vi "Main.vi"() -> ()   [LabVIEW 2019]
uses:
  Controls/Main-state.ctl
  Controls/eFGV States.ctl
  Controls/FGV States.ctl
  Controls/Global - IP Address.vi
  Controls/Global - Handle.vi
  Controls/Global - Device.vi
  Controls/Global - Comport.vi
  Controls/Global - Channel.vi
  Controls/Global - Unit.vi
  Controls/Global - Done.vi
  Controls/Global - ADC.vi
  Controls/Global - Data UDP.vi
  Controls/Global - PID.vi
  Controls/Global - System.vi
  Controls/Global - Test.vi
  Controls/UDP - Command.ctl
  <vilib>/Utility/miscctls.llb/LVRectTypeDef.ctl
  Controls/UDP - Status.ctl
  Controls/UDP - Event.ctl
  Controls/Tab Button.ctl
  <vilib>/httpClient/LabVIEWHTTPClient.lvlib
  <vilib>/httpClient/POSTBuffer.vi
panel:
  out "Close Panel":T1
  in  "Path":path
  in  "Next":bool
  in  "Previous":bool
  in  "Tab Array":T2
  out "Event":string
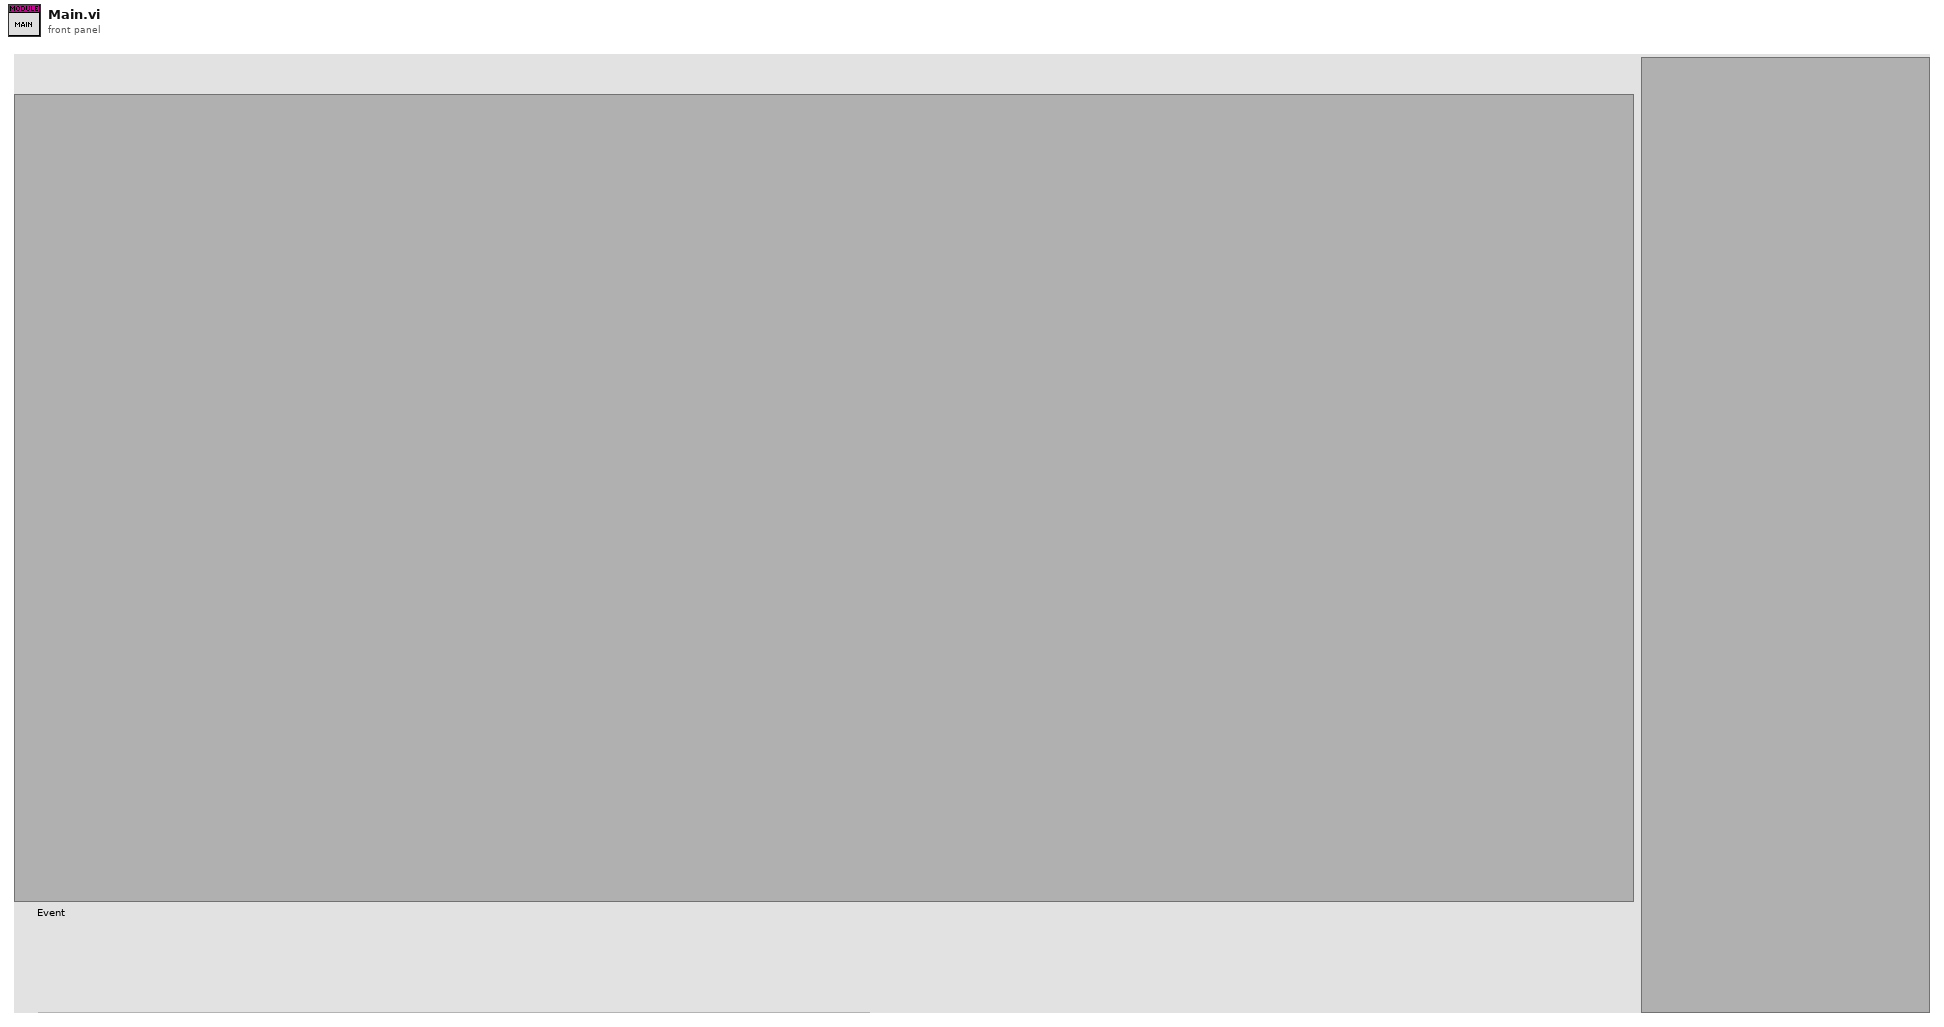
[diagram p1: front panel]
types:
  T1 = cluster{"String":string, "Cancel Button":bool, "OK Button":bool, "Bg":bool, "RunTest":refnum<vi>, "fileid":string}
  T2 = typedef "Tab Button.ctl" = cluster{"String":string, "Cancel Button":bool, "OK Button":bool, "Bg":bool, "RunTest":refnum<vi>, "fileid":string, "Stop":bool, "Run":bool, "Status":string}[]
  T3 = typedef "Main-state.ctl" = enum16{"Init", "Run modules", "Idle", "Change page", "Manual Control", "NewTest", "sidepanel", "Event", "Emergency", "Exit"}
  T4 = enum32{"Invalid", "Standard", "Closed", "Hidden", "Minimized", "Maximized"}
  T5 = enum32{"invalid app kind", "Development System", "Run Time System", "Student Edition", "Embedded LabVIEW", "Evaluation", "Custom"}
  T6 = cluster{"Module Ref":refnum<vi>[], "Side Name":string, "pin":bool, "FileId":string}
  T7 = typedef "FGV States.ctl" = enum16{"Read", "Write"}
  T8 = typedef "eFGV States.ctl" = enum16{"Init", "Read", "Write", "Exit"}
  T9 = enum16{"New Test", "Test Plan", "Job Record", "Instrument", "Machine", "Station", "Machine Control"}
  T10 = typedef "LVRectTypeDef.ctl" = cluster{"Left":i16, "Top":i16, "Right":i16, "Bottom":i16}
  T11 = typedef "UDP - Command.ctl" = enum16{"Stop", "Jog Up", "Jog Down", "Ramp Up", "Ramp Down", "PID Target", "PID Ramp", "Disp Run", "Read Ch Data", "Zero Channel", "Zero Disp", "Read Sensor", "Write Sensor", "Read ADC", "Write ADC", "Read PID", "Write PID", "Read Test", "Write Test", "Read System", "Write System", "Read Datalog", "Read Datalog Sensor"}
  T12 = cluster{"String":string, "Cancel Button":bool, "OK Button":bool, "Bg":bool, "RunTest":refnum<vi>, "fileid":string, "Stop":bool, "Run":bool, "Status":string}
  T13 = cluster{"String":string, "Cancel Button":bool, "OK Button":bool, "Bg":bool, "RunTest":refnum<vi>, "fileid":string, "Stop":bool, "Run":bool, "Status":string}[]
  T14 = typedef "LabVIEWHTTPClient.lvlib/ClientHandle.ctl" = refnum<k1>
  T15 = cluster{"IP Address":string, "port":string, "UDP ref":refnum<k16>}[]
  T16 = typedef "UDP - Event.ctl" = u16
  T17 = typedef "UDP - Status.ctl" = u16
  T18 = cluster{"Channels":cluster{"Ch1":sgl, "Ch2":sgl, "Ch3":sgl, "Ch4":sgl, "Ch5":sgl, "Ch6":sgl, "Ch7":sgl, "Ch8":sgl, "Ch9":sgl, "Ch10":sgl, "Ch11":sgl, "Ch12":sgl, "Ch13":sgl, "Ch14":sgl, "Ch15":sgl, "Ch16":sgl}, "Event":T16, "Status":T17}[]
  T19 = cluster{"Ch1":sgl, "Ch2":sgl, "Ch3":sgl, "Ch4":sgl, "Ch5":sgl, "Ch6":sgl, "Ch7":sgl, "Ch8":sgl, "Ch9":sgl, "Ch10":sgl, "Ch11":sgl, "Ch12":sgl, "Ch13":sgl, "Ch14":sgl, "Ch15":sgl, "Ch16":sgl}
  T20 = cluster{"Target Load":sgl, "Target Disp":sgl, "Rate":sgl, "Speed":sgl}[]
  T21 = cluster{"Out Type":u8, "Inverse":u8, "Monitor":u8, "Reserve":u8, "ACC Time":u32, "Pulse Rev":u32, "Stroke":u32, "Auto Off":u32, "Gear Ratio":sgl, "Pitch":sgl, "Max Speed":u32, "Jog Speed":u32, "Disp Coff":sgl, "Max Load":u32}[]
  T22 = cluster{"SP":sgl, "PV":sgl, "kP":sgl, "kI":sgl, "kD":sgl, "FF":sgl, "Err Band":sgl, "Max":i32, "Min":i32, "Ts":u32, "Out":i32, "Mode":u8}[]
  T23 = cluster{"Active Ch":u8[], "Filter Type":u8, "Post Filter":u8[], "Gain":u8[], "FS":u16, "IntOC":u8, "IntFC":u8, "SysOC":u8, "Cofficient":dbl[], "K":dbl[], "Max":i32}[]
  T24 = cluster{"Name":string[], "Unit":string[], "Decimal Point":u8[], "Ch Log":u8[], "H Alarm":u8[], "L Alarm":u8[], "H Limit":sgl[], "L Limit":sgl[], "Filter":u8[], "Gain":u8[], "Calib Type":u32[]}[]
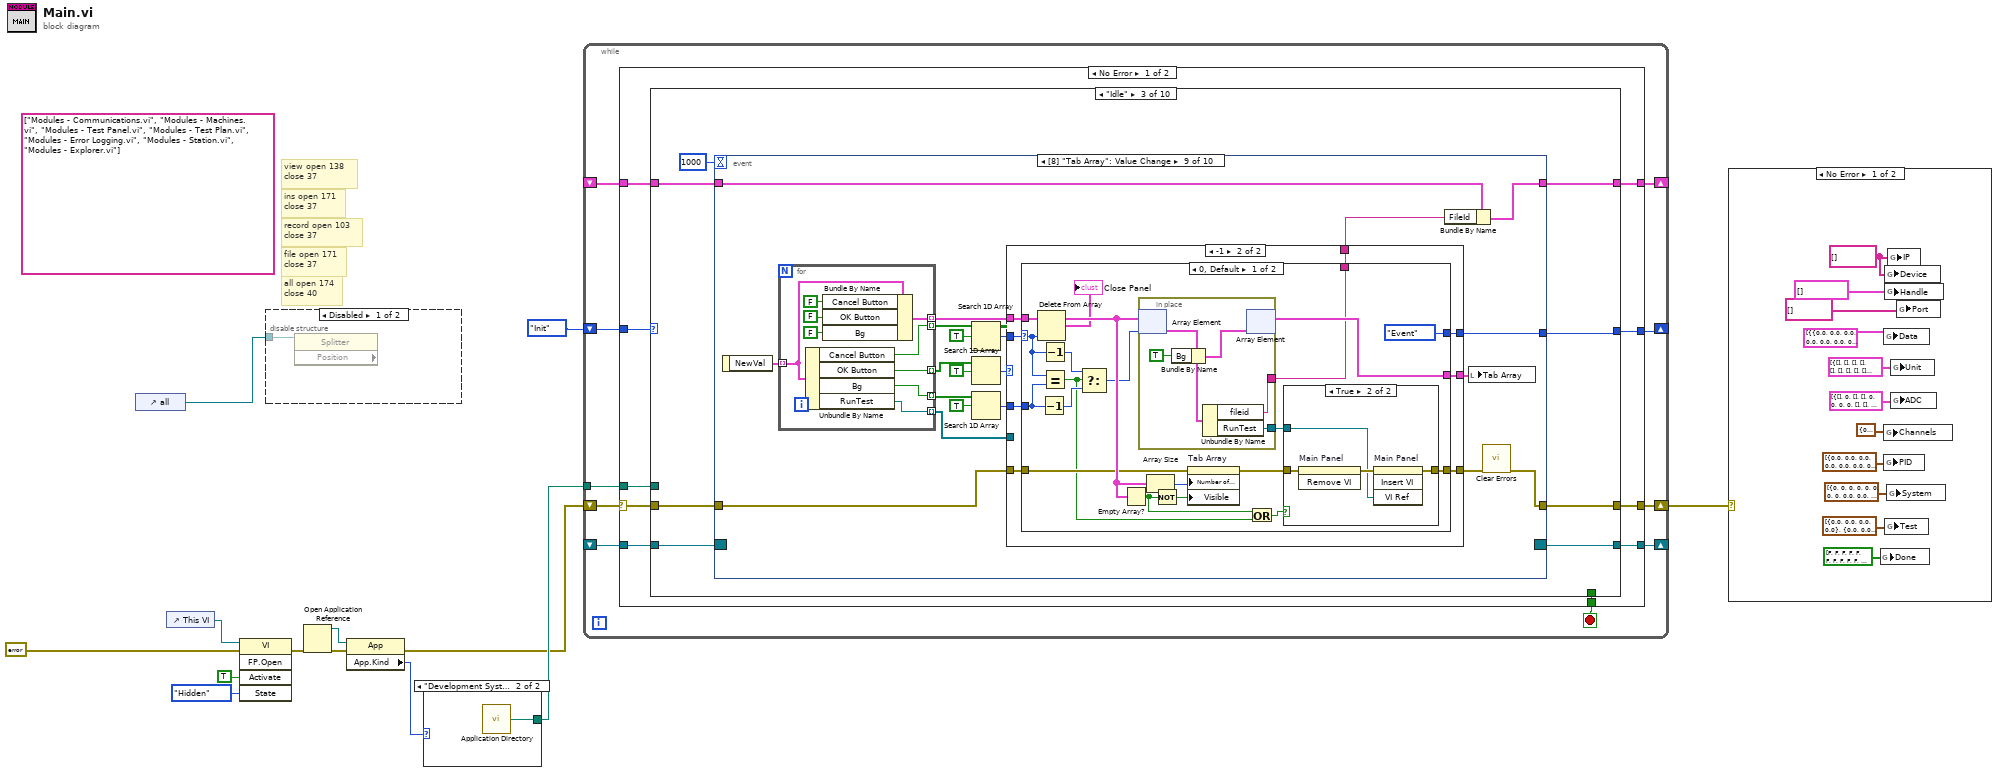
[diagram p0: block diagram]
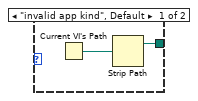
[diagram p2: hidden frame]
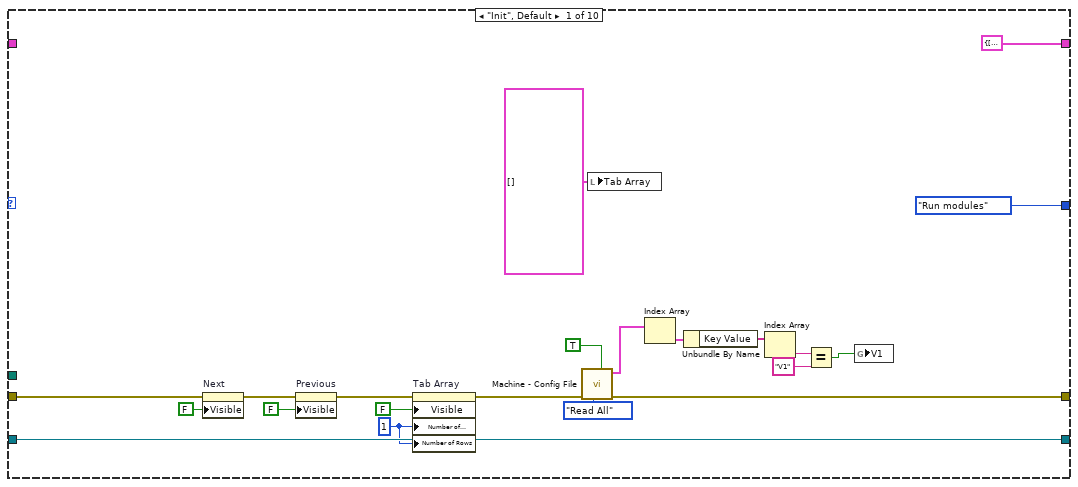
[diagram p4: hidden frame]
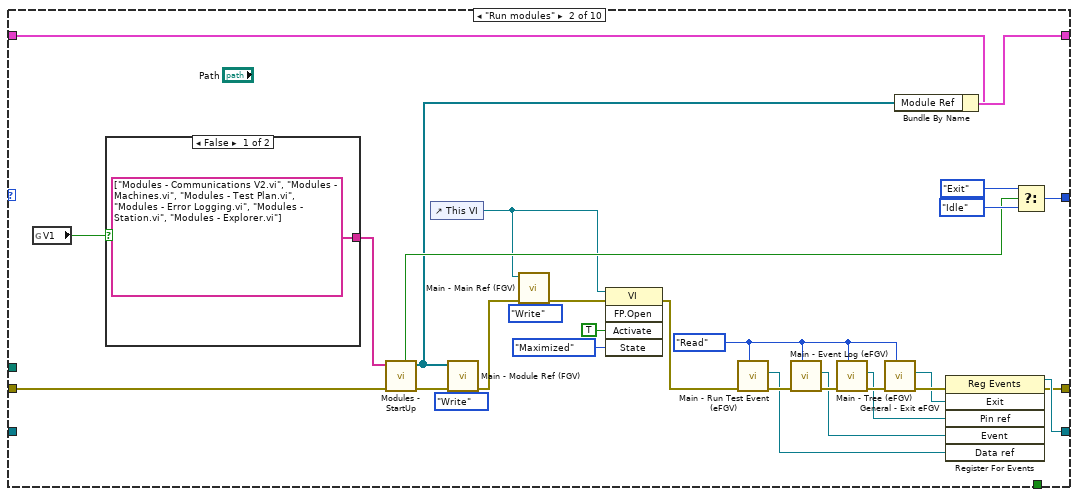
[diagram p5: hidden frame]
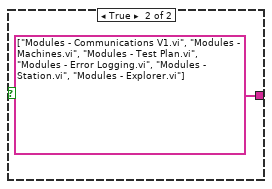
[diagram p6: hidden frame]
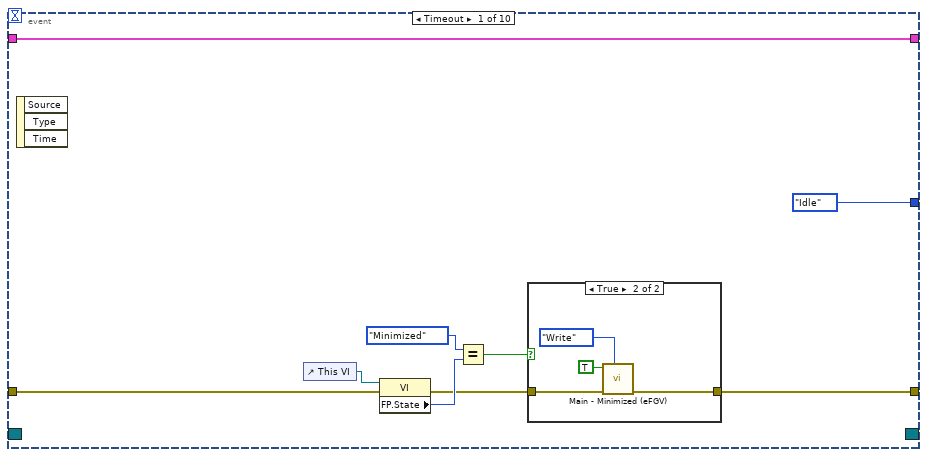
[diagram p7: hidden frame]
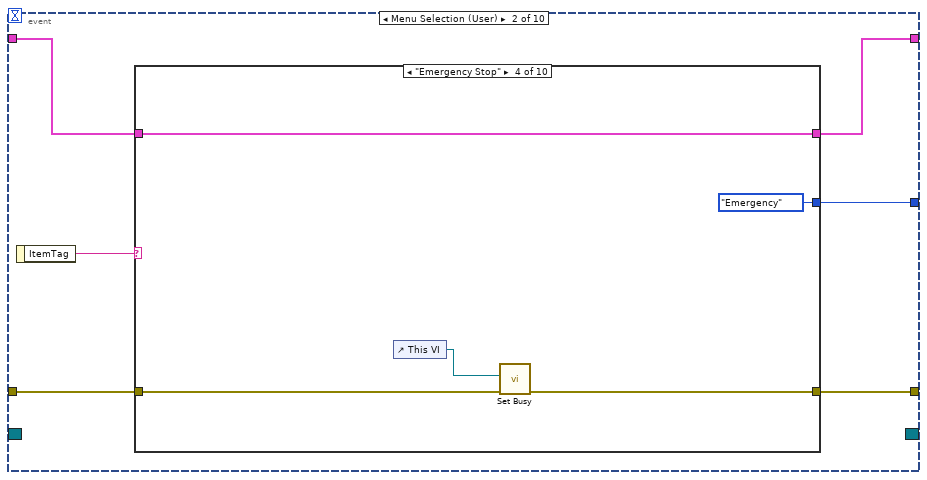
[diagram p9: hidden frame]
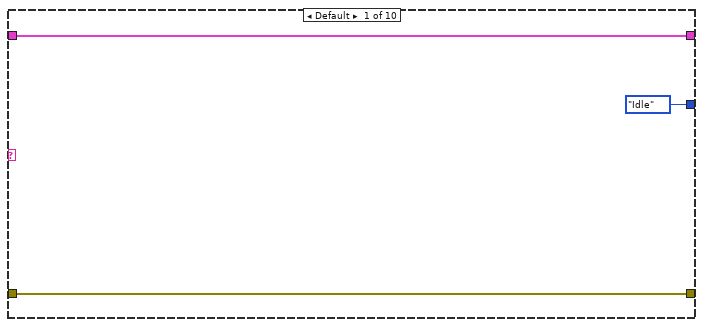
[diagram p10: hidden frame]
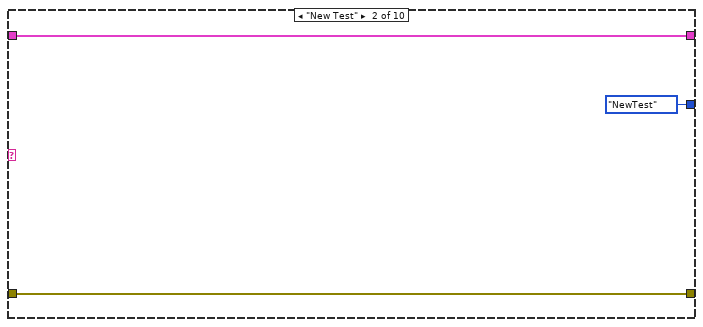
[diagram p11: hidden frame]
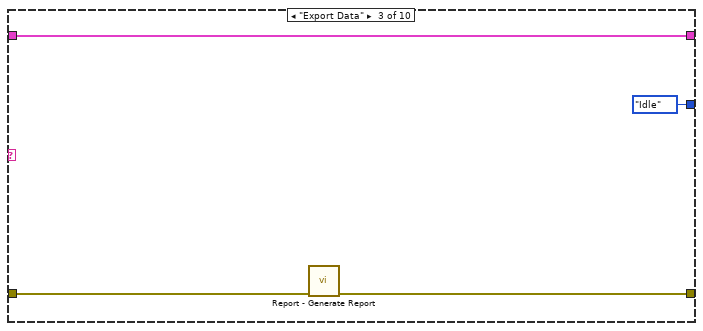
[diagram p12: hidden frame]
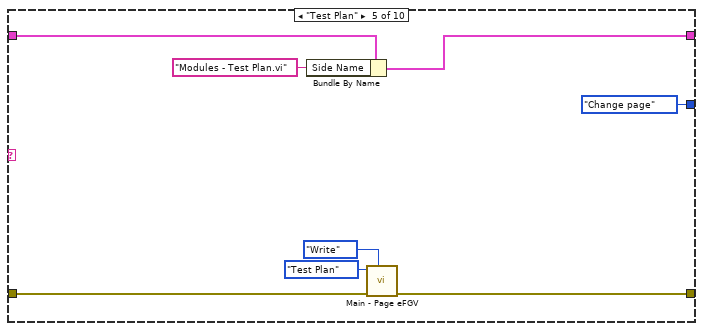
[diagram p13: hidden frame]
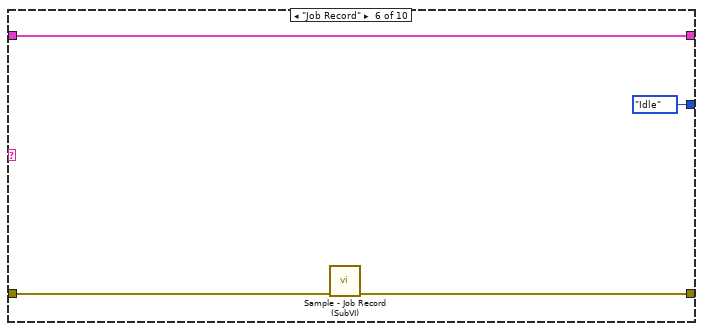
[diagram p14: hidden frame]
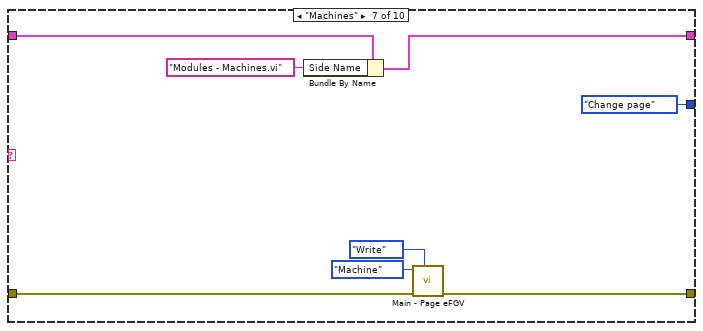
[diagram p15: hidden frame]
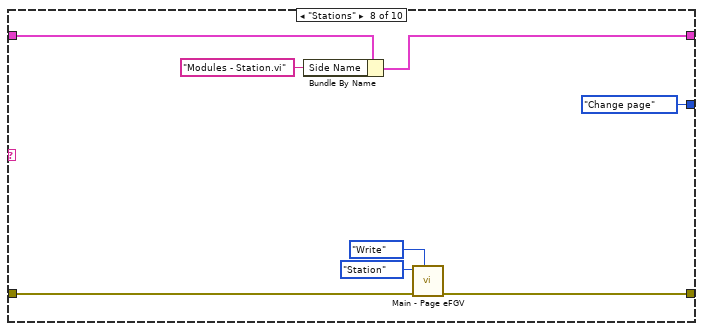
[diagram p16: hidden frame]
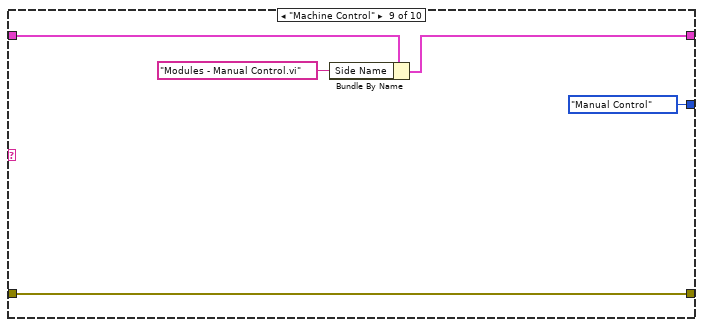
[diagram p17: hidden frame]
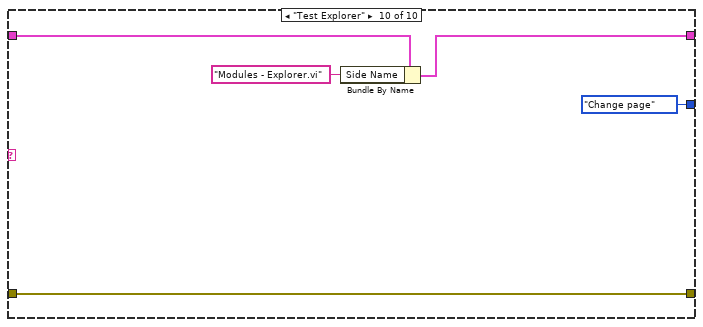
[diagram p18: hidden frame]
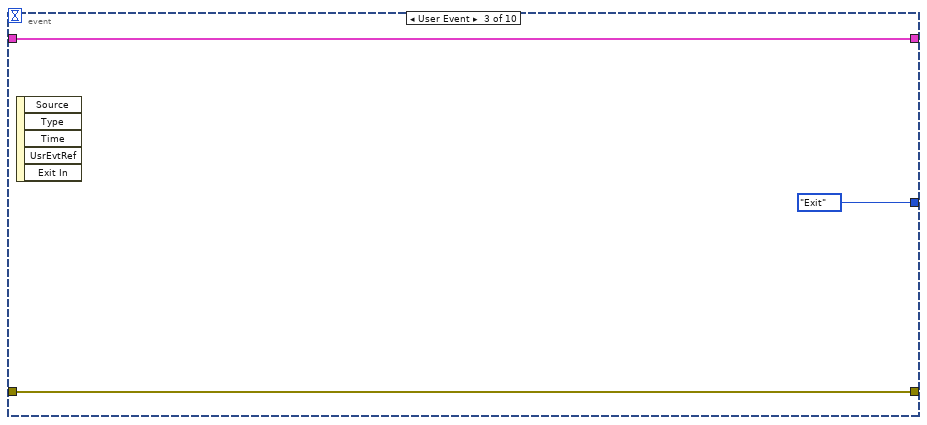
[diagram p19: hidden frame]
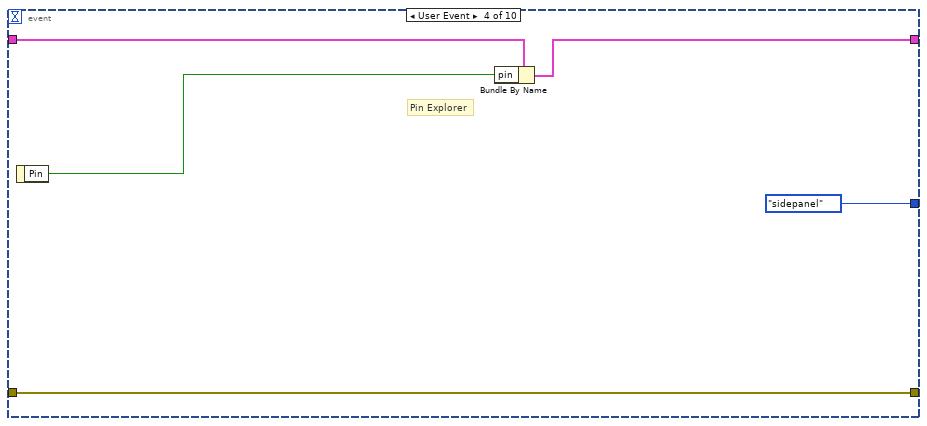
[diagram p20: hidden frame]
diagram:
  (unwired) string[] ["Modules - Communications.vi", "Modules - Machines.vi", "Modules - Test Panel.vi", "Modules - Test Plan.vi", "Modules - Error Logging.vi", "Modules - Station.vi", "Modules - Explorer.vi"]
  # "view open 138\nclose 37"
  # "record open 103\nclose 37"
  # "ins open 171\nclose 37"
  # "all open 174\nclose 40"
  # "file open 171\nclose 37"
  n1 = control-ref of="all"() -> (w1:refnum<vi>)
  n2 = control-ref of="This VI"() -> (w10:refnum<vi>)
  n3 = invoke class="VI" method="FP.Open"(reference=w10, error in=errorcluster {"status"=FALSE, "code"=0, "source"=""} ("error constant"), "Activate"=TRUE ("Activate?"), "State"=T4."Hidden") -> (error out=w5:errorcluster)  [unwired: 1 in, 4 out]
  n4 = disable-structure shown="Disabled" {
    disable-tunnel: w1 -> [w14 _]
    frame Disabled {
      n5 = property class="Splitter" props=["Position"](reference=w14) -> ()  [unwired: 1 in, 3 out]
    }
    frame Enabled {
    }
  }
  n6 = Open Application Reference(8:w5) -> (0:w7:errorcluster, 3:w6:refnum<vi>)  [unwired: 3 in]
  n7 = property class="App"(reference=w6, error in=w7) -> (error out=w2:errorcluster, "App.Kind"=w4:T5)  [unwired: 1 out]
  n8 = case shown="\"Development System\"" w4 {
    tunnel: [w15 w17] -> w3
    frame "invalid app kind", Default {
      n9 = Current VI's Path() -> (path=w16:path)
      n10 = Strip Path(path=w16) -> (stripped path=w15:path)  [unwired: 1 out]
    }
    frame "Development System" {
      n11 = call <vilib>:"Application Directory.vi"() -> ("Application Directory"=w17:path)
    }
  }
  n12 = while {
    shift-right: [w24] -> _
    shift-left: Main-state."Init" -> [w26]
    shift-right: [w25] -> w8
    shift-left: w2 -> [w27]
    shift-right: [w22] -> _
    shift-left: _ -> [w21]
    shift-right: [w20] -> _
    shift-left: _ -> [w19]
    tunnel: w3 -> [w18]
    stop <- w23 stop-if-true
    n13 = case shown="No Error" w27 {
      selector: w27 -> [w36 w640]
      tunnel: w26 -> [w37 _]
      tunnel: [w35 w637] -> w25
      tunnel: [w34 Main-state."Idle"] -> w24
      tunnel: [w33 _] -> w23
      tunnel: [w32 w639] -> w22
      tunnel: w21 -> [w31 w639]
      tunnel: [w30 w635] -> w20
      tunnel: w19 -> [w29 w635]
      tunnel: w18 -> [w28 _]
      frame No Error {
        n14 = case shown="\"Idle\"" w37 {
          tunnel: w36 -> [w53 w86 w97 w381 w415 w458 w478 w514 w575 w604]
          tunnel: [w46 w61 w98 w384 w420 w457 w481 w509 w572 w608] -> w35
          tunnel: [Main-state."Run modules" w81 w94 Main-state."Idle" Main-state."Idle" Main-state."Idle" Main-state."Idle" Main-state."Idle" Main-state."Idle" Main-state."Exit"] -> w34
          tunnel: [_ _ _ _ _ _ _ _ _ TRUE] -> w33
          tunnel: [T6 {"Module Ref"=[], "Side Name"="", "pin"=FALSE, "FileId"=""} w88 w95 w383 w424 w471 w480 w513 w577 T6 {"Module Ref"=[], "Side Name"="", "pin"=FALSE, "FileId"=""}] -> w32
          tunnel: w31 -> [_ w60 w96 w383 w424 w471 w480 w513 w577 w616]
          tunnel: [w57 w74 w91 w377 w425 w472 w483 w518 w578 w606] -> w30
          tunnel: w29 -> [w57 _ w92 w377 w425 w472 w483 w518 w578 w606]
          tunnel: w28 -> [_ _ _ _ w411 w465 _ _ _ _]
          frame "Init", Default {
            w50 = u32 1 ("Number of Columns")
            n15 = property on="Next" class="Bool"(error in=w53, "Visible"=FALSE) -> (error out=w54:errorcluster)  [unwired: 1 in, 1 out]
            n16 = property on="Previous" class="Bool"(error in=w54, "Visible"=FALSE) -> (error out=w52:errorcluster)  [unwired: 1 in, 1 out]
            n17 = property on="Tab Array" class="Arr"(error in=w52, "Visible"=FALSE, "Number of Columns"=w50, "Number of Rows"=w50) -> (error out=w47:errorcluster)  [unwired: 1 in, 1 out]
            n18 = call "Machine - Config File.vi"("Setting"=TRUE, "Action"=enum16{"Write", "Read", "Read All", "Remove"}."Read All", "error in (no error)"=w47) -> ("error out"=w46:errorcluster, "Value Out"=w42:cluster{"IP/SN":string, "Key Value":string[]}[])  [unwired: 7 in]
            n19 = local write "Tab Array"(T2 [] ("Array")) -> ()
            n20 = Index Array(array=w42) -> (element=w44:cluster{"IP/SN":string, "Key Value":string[]})  [unwired: 1 in]
            n21 = Unbundle By Name(w44) -> ("Key Value"=w43:string[])
            n22 = Index Array(array=w43) -> (element=w40:string)  [unwired: 1 in]
            n23 = Equal?(x=w40, y="V1") -> (x = y?=w38:bool)
            n24 = global write "Global - Data UDP.vi" "V1"(w38) -> ()
          }
          frame "Run modules" {
            w63 = eFGV_States."Read" ("Action")
            n25 = global read "Global - Data UDP.vi" "V1"() -> (w59:bool)
            n26 = case shown="False" w59 {
              tunnel: [string[] ["Modules - Communications V2.vi", "Modules - Machines.vi", "Modules - Test Plan.vi", "Modules - Error Logging.vi", "Modules - Station.vi", "Modules - Explorer.vi"] string[] ["Modules - Communications V1.vi", "Modules - Machines.vi", "Modules - Test Plan.vi", "Modules - Error Logging.vi", "Modules - Station.vi", "Modules - Explorer.vi"]] -> w87
              frame False {
              }
              frame True {
              }
            }
            n27 = call "Modules - StartUp.vi"("Error In"=w86, "List of Modules"=w87) -> ("Error Out"=w78:errorcluster, "Module Ref"=w77:refnum<vi>[], "Force Exit"=w80:bool)  [unwired: 7 in]
            n28 = control-ref of="This VI"() -> (w69:refnum<vi>)
            n29 = call "Main - Module Ref (FGV).vi"("Action"=FGV_States."Write", "error in"=w78, "Ref in"=w77) -> ("error out"=w71:errorcluster)  [unwired: 7 in, 1 out]
            n30 = call "Main - Main Ref (FGV).vi"("Action"=FGV_States."Write", "error in"=w71, "This VI"=w69) -> ("error out"=w70:errorcluster)  [unwired: 7 in, 1 out]
            n31 = invoke class="VI" method="FP.Open"(reference=w69, error in=w70, "Activate"=TRUE ("Activate?"), "State"=T4."Maximized") -> (error out=w65:errorcluster)  [unwired: 1 in, 4 out]
            n32 = call "Main - Run Test Event (eFGV).vi"("Action"=w63, "error in"=w65) -> ("error out"=w64:errorcluster, "Data ref"=w62:refnum<user-event>)  [unwired: 7 in, 1 out]
            n33 = call "Main - Event Log (eFGV).vi"("Action"=w63, "error in"=w64) -> ("error out"=w67:errorcluster, "Event"=w66:refnum<user-event>)  [unwired: 6 in, 2 out]
            n34 = call "Main - Tree (eFGV).vi"("Action"=w63, "error in"=w67) -> ("error out"=w73:errorcluster, "Pin ref"=w72:refnum<user-event>)  [unwired: 7 in, 1 out]
            n35 = call "General - Exit eFGV.vi"("eFGV States"=w63, "error in (no error)"=w73) -> ("error out"=w76:errorcluster, "Exit"=w75:refnum<user-event>)  [unwired: 7 in, 1 out]
            n36 = Bundle By Name(cluster=w60, "Module Ref"=w77) -> (w88:T6)
            n37 = register-events(error in=w76, w75, w72, w66, w62) -> (reference out=w74:refnum<event-registration>, error out=w61:errorcluster)  [unwired: 1 in]
            n38 = Select(t=Main-state."Exit", s=w80, f=Main-state."Idle") -> (s? t:f=w81:T3)
          }
          frame "Idle" {
            n39 = event shown="[8] \"Tab Array\": Value Change" {
              selector: w92 -> [_ _ _ _ _ _ _ _ _ _]
              dyn-events: [_ _ _ _ _ _ _ _ _ _] -> w91
              timeout: 1000 -> [_ _ _ _ _ _ _ _ _ _]
              tunnel: [w100 w118 w174 w179 w183 w186 w192 w213 w237 w324] -> w98
              tunnel: w97 -> [w104 w117 w174 w179 w183 w187 w191 w212 w240 w323]
              tunnel: w96 -> [w107 w114 w173 w176 w181 w189 w203 w224 w235 w331]
              tunnel: [w107 w113 w173 w177 w182 w189 w203 w224 w236 w331] -> w95
              tunnel: [Main-state."Idle" w115 Main-state."Exit" Main-state."sidepanel" Main-state."Event" Main-state."Exit" Main-state."Idle" Main-state."Idle" w233 Main-state."Idle"] -> w94
              event Timeout {
                n40 = event-data() -> ()  [unwired: 1 in, 3 out]
                n41 = control-ref of="This VI"() -> (w105:refnum<vi>)
                n42 = property class="VI"(reference=w105, error in=w104) -> (error out=w99:errorcluster, "FP.State"=w102:T4)  [unwired: 1 out]
                n43 = Equal?(x=T4."Minimized" ("Front Panel Window:State"), y=w102) -> (x = y?=w101:bool)
                n44 = case shown="True" w101 {
                  tunnel: [w108 w111] -> w100
                  tunnel: w99 -> [w108 w112]
                  frame False {
                  }
                  frame True {
                    n45 = call "Main - Minimized (eFGV).vi"("Action"=eFGV_States."Write", "error in"=w112, "Minimized In"=TRUE) -> ("error out"=w111:errorcluster)  [unwired: 6 in, 2 out]
                  }
                }
              }
              event Menu Selection (User) {
                n46 = event-data() -> ("ItemTag"=w116:string)  [unwired: 1 in]
                n47 = case shown="\"Emergency Stop\"" w116 {
                  tunnel: [w121 w124 w127 w131 w137 w143 w149 w157 w166 w171] -> w118
                  tunnel: w117 -> [w121 w124 w126 w130 w136 w142 w148 w156 w166 w171]
                  tunnel: [Main-state."Idle" Main-state."NewTest" Main-state."Idle" Main-state."Emergency" Main-state."Change page" Main-state."Idle" Main-state."Change page" Main-state."Change page" Main-state."Manual Control" Main-state."Change page"] -> w115
                  tunnel: [w119 w122 w125 w129 w135 w144 w147 w155 w164 w168] -> w113
                  tunnel: w114 -> [w119 w122 w125 w129 w134 w144 w146 w154 w163 w167]
                  frame Default {
                  }
                  frame "New Test" {
                  }
                  frame "Export Data" {
                    n48 = call "Report - Generate Report.vi"("error in"=w126) -> ("error out"=w127:errorcluster)  [unwired: 10 in]
                  }
                  frame "Emergency Stop" {
                    n49 = control-ref of="This VI"() -> (w132:refnum<vi>)
                    n50 = call <vilib>:"Set Busy.vi"("error in (no error)"=w130, "VI reference (current VI)"=w132) -> ("error out"=w131:errorcluster)  [unwired: 8 in, 1 out]
                  }
                  frame "Test Plan" {
                    n51 = Bundle By Name(cluster=w134, "Side Name"="Modules - Test Plan.vi") -> (w135:T6)
                    n52 = call "Main - Page eFGV.vi"("eFGV States"=eFGV_States."Write", "error in (no error)"=w136, "Page In"=T9."Test Plan") -> ("error out"=w137:errorcluster)  [unwired: 6 in, 2 out]
                  }
                  frame "Job Record" {
                    n53 = call "Sample - Job Record (SubVI).vi"("error in"=w142) -> ("error out"=w143:errorcluster)  [unwired: 10 in]
                  }
                  frame "Machines" {
                    n54 = Bundle By Name(cluster=w146, "Side Name"="Modules - Machines.vi") -> (w147:T6)
                    n55 = call "Main - Page eFGV.vi"("eFGV States"=eFGV_States."Write", "error in (no error)"=w148, "Page In"=T9."Machine") -> ("error out"=w149:errorcluster)  [unwired: 6 in, 2 out]
                  }
                  frame "Stations" {
                    n56 = Bundle By Name(cluster=w154, "Side Name"="Modules - Station.vi") -> (w155:T6)
                    n57 = call "Main - Page eFGV.vi"("eFGV States"=eFGV_States."Write", "error in (no error)"=w156, "Page In"=T9."Station") -> ("error out"=w157:errorcluster)  [unwired: 6 in, 2 out]
                  }
                  frame "Machine Control" {
                    n58 = Bundle By Name(cluster=w163, "Side Name"="Modules - Manual Control.vi") -> (w164:T6)
                  }
                  frame "Test Explorer" {
                    n59 = Bundle By Name(cluster=w167, "Side Name"="Modules - Explorer.vi") -> (w168:T6)
                  }
                }
              }
              event User Event {
                n60 = event-data() -> ()  [unwired: 1 in, 5 out]
              }
              event User Event {
                # "Pin Explorer"
                n61 = event-data() -> ("Pin"=w175:bool)  [unwired: 1 in]
                n62 = Bundle By Name(cluster=w176, "pin"=w175) -> (w177:T6)
              }
              event User Event {
                n63 = event-data() -> ("fileid"=w180:string)  [unwired: 1 in]
                n64 = Bundle By Name(cluster=w181, "FileId"=w180) -> (w182:T6)
              }
              event Panel Close? {
                n65 = event-data() -> ()  [unwired: 1 in, 4 out]
                n66 = control-ref of="This VI"() -> (w185:refnum<vi>)
                n67 = call <vilib>:"Set Busy.vi"("error in (no error)"=w187, "VI reference (current VI)"=w185) -> ("error out"=w186:errorcluster)  [unwired: 8 in, 1 out]
                n68 = event-data("Discard?"=TRUE) -> ()  [unwired: 1 in, 1 out]
              }
              event "Previous": Value Change {
                n69 = event-data() -> ()  [unwired: 1 in, 1 out]
                n70 = property on="Tab Array" class="Arr"(error in=w191) -> (error out=w194:errorcluster, "Index Values"=w201:u32[], "Number of Columns"=w198:u32)  [unwired: 1 in, 1 out]
                n71 = Subtract(x=w198, y=u32 12) -> (x-y=w196:u32)
                n72 = Increment(x=w201) -> (x+1=w195:u32[])
                n73 = Index Array(array=w195) -> (element=w200:u32)  [unwired: 1 in]
                n74 = property on="Tab Array" class="Arr"(error in=w194, "Index Values"=w195) -> (error out=w193:errorcluster)  [unwired: 1 in, 1 out]
                n75 = Equal?(x=w196, y=w200) -> (x = y?=w199:bool)
                n76 = case shown="True" w199 {
                  tunnel: w193 -> [w205 w209]
                  tunnel: [w204 w207] -> w192
                  frame False {
                    n77 = property on="Next" class="Bool"(error in=w205, "Visible"=TRUE) -> (error out=w204:errorcluster)  [unwired: 1 in, 1 out]
                  }
                  frame True {
                    n78 = property on="Next" class="Bool"(error in=w209, "Visible"=TRUE) -> (error out=w208:errorcluster)  [unwired: 1 in, 1 out]
                    n79 = property on="Previous" class="Bool"(error in=w208, "Visible"=FALSE) -> (error out=w207:errorcluster)  [unwired: 1 in, 1 out]
                  }
                }
              }
              event "Next": Value Change {
                n80 = event-data() -> ()  [unwired: 1 in, 1 out]
                n81 = property on="Tab Array" class="Arr"(error in=w212) -> (error out=w215:errorcluster, "Index Values"=w222:u32[], "Number of Columns"=w219:u32)  [unwired: 1 in, 1 out]
                n82 = Subtract(x=w219, y=u32 12) -> (x-y=w217:u32)
                n83 = Increment(x=w222) -> (x+1=w216:u32[])
                n84 = Index Array(array=w216) -> (element=w221:u32)  [unwired: 1 in]
                n85 = property on="Tab Array" class="Arr"(error in=w215, "Index Values"=w216) -> (error out=w214:errorcluster)  [unwired: 1 in, 1 out]
                n86 = Equal?(x=w217, y=w221) -> (x = y?=w220:bool)
                n87 = case shown="True" w220 {
                  tunnel: w214 -> [w226 w231]
                  tunnel: [w225 w228] -> w213
                  frame False {
                    n88 = property on="Previous" class="Bool"(error in=w226, "Visible"=TRUE) -> (error out=w225:errorcluster)  [unwired: 1 in, 1 out]
                  }
                  frame True {
                    n89 = property on="Previous" class="Bool"(error in=w231, "Visible"=TRUE) -> (error out=w229:errorcluster)  [unwired: 1 in, 1 out]
                    n90 = property on="Next" class="Bool"(error in=w229, "Visible"=FALSE) -> (error out=w228:errorcluster)  [unwired: 1 in, 1 out]
                  }
                }
              }
              event Value Change {
                n91 = event-data() -> ("NewVal"=w242:T2)  [unwired: 1 in]
                n92 = for {
                  tunnel: w242 -> [w315] mode=indexing
                  tunnel: [w317] -> w243 mode=indexing
                  tunnel: [w316] -> w246 mode=indexing
                  tunnel: [w312] -> w248 mode=indexing
                  tunnel: [w310] -> w251 mode=indexing
                  tunnel: [w309] -> w238 mode=indexing
                  n93 = Unbundle By Name(w315) -> ("Cancel Button"=w317:bool, "OK Button"=w316:bool, "Bg"=w310:bool, "RunTest"=w309:refnum<vi>)
                  n94 = Bundle By Name(cluster=w315, "Cancel Button"=FALSE, "OK Button"=FALSE, "Bg"=FALSE) -> (w312:T12)
                }
                n95 = Search 1D Array(1D array=w243, element=TRUE) -> (index of element=w247:i32)  [unwired: 1 in]
                n96 = Search 1D Array(1D array=w246, element=TRUE) -> (index of element=w249:i32)  [unwired: 1 in]
                n97 = Search 1D Array(1D array=w251, element=TRUE) -> (index of element=w252:i32)  [unwired: 1 in]
                n98 = case shown="-1" w249 {
                  selector: w249 -> [w257 _]
                  tunnel: w247 -> [_ w274]
                  tunnel: w248 -> [w262 w273]
                  tunnel: [w261 w272] -> w241
                  tunnel: w252 -> [_ w271]
                  tunnel: w240 -> [w259 w270]
                  tunnel: [w260 w269] -> w239
                  tunnel: w238 -> [w258 _]
                  tunnel: [w255 w268] -> w234
                  tunnel: [Main-state."Event" w267] -> w233
                  frame 0, Default {
                    # "Open Sub Panel"
                    n99 = in-place {
                      in-place-border: [w263] -> w255
                      n100 = in-place-array #1(w262, w257) -> (w266:T12)
                      n101 = Bundle By Name(cluster=w266, "Bg"=TRUE) -> (w264:T12)
                      n102 = Unbundle By Name(w264) -> ("fileid"=w263:string)
                      n103 = in-place-array #1(w264) -> (w261:T13)  [unwired: 1 out]
                    }
                    n104 = Index Array(array=w258, index=w257) -> (element=w256:refnum<vi>)
                    n105 = invoke on="Main Panel" class="SubPnl" method="Insert VI"(error in=w259, "VI Ref"=w256) -> (error out=w260:errorcluster)  [unwired: 2 in, 3 out]
                    n106 = local write "Close Panel"(T1 {"String"="", "Cancel Button"=FALSE, "OK Button"=FALSE, "Bg"=FALSE, "RunTest"=refnum, "fileid"=""} ("Close Panel")) -> ()
                  }
                  frame -1 {
                    n107 = case shown="0, Default" w274 {
                      selector: w274 -> [w292 _]
                      tunnel: w273 -> [w294 w308]
                      tunnel: [w293 w308] -> w272
                      tunnel: w271 -> [w289 _]
                      tunnel: w270 -> [w285 w307]
                      tunnel: [w283 w307] -> w269
                      tunnel: [w277 "" ("fileid")] -> w268
                      tunnel: [Main-state."Event" Main-state."Idle"] -> w267
                      frame 0, Default {
                        n108 = Delete From Array(array=w294, index=w292) -> (deleted portion=→"Close Panel":T12, array with subset deleted=w291:T13)  [unwired: 1 in]
                        n109 = Decrement(x=w289) -> (x-1=w288:i32)
                        n110 = Decrement(x=w292) -> (x-1=w290:i32)
                        n111 = Equal?(x=w292, y=w289) -> (x = y?=w280:bool)
                        n112 = Select(t=w290, s=w280, f=w288) -> (s? t:f=w282:i32)
                        n113 = Empty Array?(array=w291) -> (empty?=w279:bool)
                        n114 = in-place {
                          in-place-border: [w301] -> w281
                          in-place-border: [w300] -> w277
                          n115 = in-place-array #2(w291, w282) -> (w304:T12)
                          n116 = Bundle By Name(cluster=w304, "Bg"=TRUE) -> (w302:T12)
                          n117 = Unbundle By Name(w302) -> ("fileid"=w300:string, "RunTest"=w301:refnum<vi>)
                          n118 = in-place-array #2(w302) -> (w293:T13)  [unwired: 1 out]
                        }
                        n119 = Array Size(array=w291) -> (size(s)=w287:i32)
                        n120 = Not(x=w279) -> (.not. x?=w286:bool)
                        n121 = property on="Tab Array" class="Arr"(error in=w285, "Number of Columns"=w287, "Visible"=w286) -> (error out=w284:errorcluster)  [unwired: 1 in, 1 out]
                        n122 = Or(x=w279, y=w280) -> (x .or. y?=w278:bool)
                        n123 = case shown="True" w278 {
                          tunnel: w284 -> [w295 w299]
                          tunnel: [w295 w297] -> w283
                          tunnel: w281 -> [_ w296]
                          frame False {
                          }
                          frame True {
                            n124 = invoke on="Main Panel" class="SubPnl" method="Remove VI"(error in=w299) -> (error out=w298:errorcluster)  [unwired: 2 in, 2 out]
                            n125 = invoke on="Main Panel" class="SubPnl" method="Insert VI"(error in=w298, "VI Ref"=w296) -> (error out=w297:errorcluster)  [unwired: 2 in, 3 out]
                          }
                        }
                      }
                      frame -1 {
                      }
                    }
                  }
                }
                n126 = Bundle By Name(cluster=w235, "FileId"=w234) -> (w236:T6)
                n127 = local write "Tab Array"(w241) -> ()
                n128 = call <vilib>:"Clear Errors.vi"("error in (no error)"=w239) -> ("error out"=w237:errorcluster)  [unwired: 5 in, 1 out]
              }
              event User Event {
                n129 = event-data() -> ("RunTest"=w322:refnum<vi>, "Name"=w319:string, "FileId"=w318:string)  [unwired: 1 in]
                n130 = Empty Array?(array="Tab Array") -> (empty?=w326:bool)
                n131 = for {
                  tunnel: "Tab Array" -> [w364] mode=indexing
                  tunnel: [w366] -> w328 mode=indexing
                  tunnel: [w363] -> w321 mode=indexing
                  n132 = Unbundle By Name(w364) -> ("RunTest"=w363:refnum<vi>)
                  n133 = Bundle By Name(cluster=w364, "Cancel Button"=FALSE, "OK Button"=FALSE, "Bg"=FALSE) -> (w366:T12)
                }
                n134 = case shown="False" w326 {
                  tunnel: [w370 0] -> w327
                  tunnel: "Tab Array" -> [w371 _]
                  tunnel: [w369 w372] -> w329
                  tunnel: w323 -> [w369 _]
                  frame False {
                    n135 = Array Size(array=w371) -> (size(s)=w370:i32)
                  }
                  frame True {
                    n136 = property on="Tab Array" class="Arr"("Visible"=TRUE) -> (error out=w372:errorcluster)  [unwired: 2 in, 1 out]
                  }
                }
                n137 = Search 1D Array(1D array=w321, element=w322) -> (index of element=w320:i32)  [unwired: 1 in]
                n138 = case shown="-1" w320 {
                  selector: w320 -> [w336 _]
                  tunnel: w329 -> [w334 w358]
                  tunnel: w328 -> [w337 w354]
                  tunnel: w327 -> [_ w349]
                  tunnel: [w333 w350] -> w324
                  tunnel: w322 -> [_ w345]
                  tunnel: w319 -> [w332 w348]
                  tunnel: w318 -> [_ w344]
                  frame 0, Default {
                    n139 = in-place {
                      in-place-border: w332 -> [w339]
                      n140 = in-place-array #3(w337, w336) -> (w342:T12)
                      n141 = Bundle By Name(cluster=w342, "OK Button"=TRUE, "Bg"=TRUE, "String"=w339) -> (w340:T12)
                      n142 = in-place-array #3(w340) -> (w335:T13)  [unwired: 1 out]
                    }
                    n143 = property on="Tab Array" class="Arr"(error in=w334, "Val(Sgnl)"=w335) -> (error out=w333:errorcluster)  [unwired: 1 in, 1 out]
                  }
                  frame -1 {
                    w351 = 12 ("y")
                    n144 = Increment(x=w349) -> (x+1=w356:i32)
                    n145 = Greater?(x=w356, y=w351) -> (0:w352:bool)
                    n146 = Subtract(x=w356, y=w351) -> (x-y=w353:i32)
                    n147 = Bundle By Name(cluster=T1 {"String"="", "Cancel Button"=FALSE, "OK Button"=TRUE, "Bg"=TRUE, "RunTest"=refnum, "fileid"=""} ("new element/subarray"), "RunTest"=w345, "String"=w348, "fileid"=w344) -> (w346:T1)
                    n148 = Build Array(w353) -> (w355:i32[])
                    n149 = property on="Tab Array" class="Arr"(error in=w358, "Number of Columns"=w356, "Index Values"=w355) -> (error out=w357:errorcluster)  [unwired: 1 in, 1 out]
                    n150 = Insert Into Array(array=w354, index=w349, new element=w346) -> (w343:T13)
                    n151 = case shown="True" w352 {
                      tunnel: w357 -> [w359 w361]
                      tunnel: [w359 w360] -> w350
                      frame False {
                      }
                      frame True {
                        n152 = property on="Previous" class="Bool"(error in=w361, "Visible"=TRUE) -> (error out=w360:errorcluster)  [unwired: 1 in, 1 out]
                      }
                    }
                    n153 = property on="Tab Array" class="Arr"("Val(Sgnl)"=w343) -> ()  [unwired: 2 in, 2 out]
                  }
                }
              }
            }
          }
          frame "Change page" {
            n154 = Unbundle By Name(w383) -> ("Module Ref"=w378:refnum<vi>[], "Side Name"=w375:string)
            n155 = call "Main - Search VI Ref (SubVI).vi"("Error In"=w381, "VI Name to Search"=w375, "VI Refs"=w378) -> ("Error Out"=w380:errorcluster, "VI Ref Found"=w376:refnum<vi>, "Found?"=w379:bool)  [unwired: 6 in]
            n156 = case shown="\"Modules - Explorer.vi\"" w375 {
              tunnel: [w389 w399] -> w385
              tunnel: w380 -> [w388 w398]
              tunnel: w379 -> [w387 w397]
              tunnel: w376 -> [w386 w396]
              frame Default {
                n157 = case shown="True" w387 {
                  tunnel: [w390 w393] -> w389
                  tunnel: w386 -> [_ w392]
                  tunnel: w388 -> [w390 w391]
                  frame False {
                  }
                  frame True {
                    n158 = invoke class="VI" method="FP.Open"(reference=w392, error in=w391, "Activate"=TRUE ("Activate?"), "State"=T4."Standard") -> (error out=w393:errorcluster)  [unwired: 1 in, 4 out]
                  }
                }
              }
              frame "Modules - Explorer.vi" {
                n159 = case shown="True" w397 {
                  tunnel: [w400 w407] -> w399
                  tunnel: w396 -> [_ w402]
                  tunnel: w398 -> [w400 w406]
                  frame False {
                  }
                  frame True {
                    n160 = invoke on="Sub Panel" class="SubPnl" method="Remove VI"(error in=w406) -> (error out=w404:errorcluster)  [unwired: 2 in, 2 out]
                    n161 = property class="VI"(reference=w402, error in=w404, "Front Panel.WinBounds"=T10 {"Left"=1146, "Top"=168, "Right"=1492, "Bottom"=898} ("Front Panel Window:Window Bounds")) -> (reference out=w403:refnum<vi>, error out=w401:errorcluster)
                    n162 = invoke class="VI" method="FP.Open"(reference=w403, error in=w401, "Activate"=TRUE ("Activate?"), "State"=T4."Standard") -> (error out=w407:errorcluster)  [unwired: 1 in, 4 out]
                  }
                }
              }
            }
            n163 = call <vilib>:"Clear Errors.vi"("error in (no error)"=w385) -> ("error out"=w384:errorcluster)  [unwired: 5 in, 1 out]
          }
          frame "Manual Control" {
            (unwired) "Modules - Manual Control-ausie.vit"
            w416 = "Main" ("element")
            n164 = call "Main - Manual Control Deamon Ref (FGV).vi"("Action"=FGV_States."Read", "error in"=w415) -> ("error out"=w422:errorcluster, "Name out"=w417:string[], "Ref out"=w418:refnum<vi>[])  [unwired: 7 in]
            n165 = Build Path(base path=w411, name or relative path="Modules") -> (appended path=w414:path)
            n166 = Search 1D Array(1D array=w417, element=w416) -> (index of element=w419:i32)  [unwired: 1 in]
            n167 = Build Path(base path=w414, name or relative path="Modules - Manual Control.vit") -> (appended path=w412:path)
            n168 = case shown="0, Default" w419 {
              selector: w419 -> [w431 _]
              tunnel: w422 -> [w430 w454]
              tunnel: [w429 w449] -> w420
              tunnel: w418 -> [w432 w445]
              tunnel: w417 -> [_ w448]
              tunnel: w416 -> [_ w447]
              tunnel: w412 -> [_ w437]
              frame 0, Default {
                n169 = Index Array(array=w432, index=w431) -> (element=w428:refnum<vi>)
                n170 = invoke class="VI" method="FP.Open"(reference=w428, error in=w430, "Activate"=TRUE ("Activate?"), "State"=T4."Standard") -> (error out=w429:errorcluster)  [unwired: 1 in, 4 out]
              }
              frame -1 {
                n171 = Open VI Reference(vi path=w437, error in (no error)=w454) -> (vi reference=w453:refnum<vi>, error out=w452:errorcluster)  [unwired: 4 in]
                n172 = Build Array (concatenate)(w448, w447) -> (w444:string[])
                n173 = invoke class="VI" method="Ctrl Val.Set"(reference=w453, error in=w452, "Control Name"="Device Name", "Value"="" ("Control Name")) -> (reference out=w436:refnum<vi>, error out=w434:errorcluster)  [unwired: 1 in, 3 out]
                n174 = invoke class="VI" method="Run VI"(reference=w436, error in=w434, "Wait until done"=FALSE ("Wait Until Done"), "Auto Dispose Ref"=FALSE ("Auto Dispose Reference")) -> (reference out=w435:refnum<vi>, error out=w433:errorcluster)  [unwired: 1 in, 3 out]
                n175 = invoke class="VI" method="FP.Open"(reference=w435, error in=w433, "Activate"=TRUE ("Activate?"), "State"=T4."Standard") -> (error out=w441:errorcluster)  [unwired: 1 in, 4 out]
                n176 = Build Array (concatenate)(w445, w435) -> (w446:refnum<vi>[])
                n177 = call "Main - Manual Control Deamon Ref (FGV).vi"("Action"=FGV_States."Write", "error in"=w441, "Name"=w444, "Ref in"=w446) -> ("error out"=w449:errorcluster)  [unwired: 5 in, 2 out]
              }
            }
          }
          frame "NewTest" {
            n178 = Build Path(base path=w465, name or relative path="Modules") -> (appended path=w469:path)
            n179 = Build Path(base path=w469, name or relative path="Modules - Run Test with Config.vit") -> (appended path=w466:path)
            n180 = Open VI Reference(vi path=w466, error in (no error)=w458) -> (vi reference=w456:refnum<vi>, error out=w455:errorcluster)  [unwired: 4 in]
            n181 = invoke class="VI" method="Run VI"(reference=w456, error in=w455, "Wait until done"=FALSE ("Wait Until Done"), "Auto Dispose Ref"=FALSE ("Auto Dispose Reference")) -> (reference out=w460:refnum<vi>, error out=w459:errorcluster)  [unwired: 1 in, 3 out]
            n182 = invoke class="VI" method="FP.Open"(reference=w460, error in=w459, "Activate"=TRUE ("Activate?"), "State"=T4."Standard") -> (error out=w457:errorcluster)  [unwired: 1 in, 4 out]
          }
          frame "sidepanel" {
            n183 = Unbundle By Name(w480) -> ("Module Ref"=w477:refnum<vi>[], "pin"=w473:bool)
            n184 = call "Main - Search VI Ref (SubVI).vi"("Error In"=w478, "VI Name to Search"="Modules - Explorer.vi", "VI Refs"=w477) -> ("Error Out"=w479:errorcluster, "VI Ref Found"=w475:refnum<vi>, "Found?"=w474:bool)  [unwired: 6 in]
            n185 = case shown="True" w473 {
              tunnel: [w487 w495] -> w481
              tunnel: w479 -> [w486 w494]
              tunnel: w475 -> [w485 w492]
              tunnel: w474 -> [w484 w493]
              frame True {
                n186 = case shown="True" w484 {
                  tunnel: [w488 w491] -> w487
                  tunnel: w486 -> [w488 w490]
                  tunnel: w485 -> [_ w489]
                  frame False {
                  }
                  frame True {
                    n187 = invoke on="Sub Panel" class="SubPnl" method="Insert VI"(error in=w490, "VI Ref"=w489) -> (error out=w491:errorcluster)  [unwired: 2 in, 3 out]
                  }
                }
              }
              frame False {
                n188 = case shown="True" w493 {
                  tunnel: [w496 w504] -> w495
                  tunnel: w494 -> [w496 w505]
                  tunnel: w492 -> [_ w499]
                  frame False {
                  }
                  frame True {
                    n189 = invoke on="Sub Panel" class="SubPnl" method="Remove VI"(error in=w505) -> (error out=w498:errorcluster)  [unwired: 2 in, 2 out]
                    n190 = property class="VI"(reference=w499, error in=w498, "Front Panel.WinBounds"=T10 {"Left"=1146, "Top"=168, "Right"=1492, "Bottom"=898} ("Front Panel Window:Window Bounds")) -> (reference out=w500:refnum<vi>, error out=w497:errorcluster)
                    n191 = invoke class="VI" method="FP.Open"(reference=w500, error in=w497, "Activate"=TRUE ("Activate?"), "State"=T4."Standard") -> (error out=w504:errorcluster)  [unwired: 1 in, 4 out]
                  }
                }
              }
            }
          }
          frame "Event" {
            n192 = Unbundle By Name(w513) -> ("FileId"=w512:string)
            n193 = local read "Close Panel"() -> (w511:T1)
            n194 = call "Main - Event Log (eFGV).vi"("Action"=eFGV_States."Read", "error in"=w514, "Fileid"=w512) -> ("error out"=w508:errorcluster, "Data Out"=→"Event":string)  [unwired: 5 in, 2 out]
            n195 = Unbundle By Name(w511) -> ("fileid"=w506:string, "RunTest"=w507:refnum<vi>)
            n196 = Empty String/Path?(string/path=w506) -> (empty?=w510:bool)
            n197 = case shown="False" w510 {
              tunnel: [w525 w570] -> w509
              tunnel: w508 -> [w536 w570]
              tunnel: w507 -> [w519 _]
              tunnel: w506 -> [w528 _]
              frame False {
                n198 = property class="VI"(reference=w519, error in=w536) -> (error out=w535:errorcluster, "Front Panel.Title"=w522:string)  [unwired: 1 out]
                n199 = Search and Replace String(input string=w522, search string="Complete") -> (number of replacements=w521:i32)  [unwired: 6 in, 3 out]
                n200 = Search and Replace String(input string=w522, search string="Idle", error in=w535) -> (number of replacements=w533:i32, error out=w527:errorcluster)  [unwired: 5 in, 2 out]
                n201 = Bundle By Name(cluster=cluster{"action":string, "id":string} {"action"="delete", "id"=""}, "id"=w528) -> (w526:cluster{"action":string, "id":string})
                n202 = Greater Than 0?(x=w521) -> (x > 0?=w520:bool)
                n203 = Greater Than 0?(x=w533) -> (x > 0?=w524:bool)
                n204 = case shown="False" w524 {
                  tunnel: "http://localhost/filename.php" ("url") -> [_ w569]
                  tunnel: "Content-Type" ("header") -> [_ w566]
                  tunnel: "application/json" ("value") -> [_ w565]
                  tunnel: w527 -> [w539 w562]
                  tunnel: w526 -> [_ w560]
                  tunnel: [w538 w554] -> w525
                  tunnel: w520 -> [w540 _]
                  tunnel: w519 -> [w537 _]
                  frame False {
                    n205 = case shown="True" w540 {
                      tunnel: w539 -> [w541 w550]
                      tunnel: [w541 w543] -> w538
                      tunnel: w537 -> [_ w542]
                      frame False {
                      }
                      frame True {
                        n206 = call "Runtest - Deamon Ref (FGV).vi"("Action"=FGV_States."Read", "error in"=w550) -> ("error out"=w551:errorcluster, "Name out"=w548:string[], "Ref out"=w549:refnum<vi>[])  [unwired: 7 in]
                        n207 = Search 1D Array(1D array=w549, element=w542) -> (index of element=w547:i32)  [unwired: 1 in]
                        n208 = Delete From Array(array=w549, index=w547) -> (array with subset deleted=w545:refnum<vi>[])  [unwired: 1 in, 1 out]
                        n209 = Delete From Array(array=w548, index=w547) -> (array with subset deleted=w546:string[])  [unwired: 1 in, 1 out]
                        n210 = call "Runtest - Deamon Ref (FGV).vi"("Action"=FGV_States."Write", "error in"=w551, "Name"=w546, "Ref in"=w545) -> ("error out"=w544:errorcluster)  [unwired: 5 in, 2 out]
                        n211 = invoke class="VI" method="Abort VI"(reference=w542, error in=w544) -> (error out=w543:errorcluster)  [unwired: 1 in, 2 out]
                      }
                    }
                  }
                  frame True {
                    n212 = Flatten To JSON(anything=w560, error in (no error)=w562) -> (JSON string=w559:string, 11:w561:errorcluster)  [unwired: 1 in]
                    n213 = call <vilib>:"OpenHandle.vi"("error in (no error)"=w561) -> ("client handle out"=w567:T14, "error out"=w568:errorcluster)  [unwired: 13 in]
                    n214 = call <vilib>:"AddHeader.vi"("client handle"=w567, "header"=w566, "value"=w565, "error in (no error)"=w568) -> ("client handle out"=w563:T14, "error out"=w564:errorcluster)  [unwired: 10 in]
                    n215 = call-poly <vilib>:"POST.vi"("client handle"=w563, "url"=w569, "buffer"=w559, "error in (no error)"=w564) -> ("client handle out"=w557:T14, "error out"=w558:errorcluster)  [unwired: 8 in, 2 out]
                    n216 = call <vilib>:"CloseHandle.vi"("client handle"=w557, "error in (no error)"=w558) -> ("error out"=w555:errorcluster)  [unwired: 13 in]
                    n217 = call "Main - Update Tree (eFGV).vi"("Action"=eFGV_States."Write", "error in"=w555) -> ("error out"=w554:errorcluster)  [unwired: 7 in, 2 out]
                  }
                }
              }
              frame True {
              }
            }
          }
          frame "Emergency" {
            n218 = local read "Tab Array"() -> (w576:T2)
            n219 = for {
              tunnel: w576 -> [w594] mode=indexing
              shift-right: [w592] -> w573
              shift-left: w575 -> [w591]
              n220 = Unbundle By Name(w594) -> ("fileid"=w588:string)
              n221 = Concatenate Strings("Emergency", " - " ("string"), w588) -> (w587:string)
              n222 = call "Main - EndStage (eFGV).vi"("Action"=eFGV_States."Write", "error in"=w591, "Endstage In"=w587) -> ("error out"=w592:errorcluster)  [unwired: 6 in, 2 out]
            }
            n223 = global read "Global - IP Address.vi" "IP"() -> (w571:string[])
            n224 = for {
              shift-right: [w580] -> w572
              shift-left: w573 -> [w581]
              tunnel: w571 -> [w579] mode=indexing
              n225 = case shown="\"True\", Default" w579 {
                selector: w579 -> [_ w583]
                tunnel: w581 -> [w582 w585]
                tunnel: [w582 w584] -> w580
                frame "" {
                }
                frame "True", Default {
                  n226 = call "Communication - Send Command Read.vi"("error in (no error)"=w585, "Action"=UDP_-_Command."Stop", "Device IP Address"=w583) -> ("error out"=w584:errorcluster)  [unwired: 8 in]
                }
              }
            }
          }
          frame "Exit" {
            n227 = Unbundle By Name(w616) -> ("Module Ref"=w613:refnum<vi>[])
            n228 = global read "Global - IP Address.vi" "IP"() -> (w603:string[])
            n229 = for {
              tunnel: w603 -> [w628] mode=indexing
              shift-right: [w630] -> w602
              shift-left: w604 -> [w629]
              n230 = call "Communication - Send Command Read.vi"("Bypass?"=FALSE, "error in (no error)"=w629, "Action"=UDP_-_Command."Stop", "Device IP Address"=w628) -> ("error out"=w630:errorcluster)  [unwired: 7 in]
            }
            n231 = global read "Global - Handle.vi" "Handle"() -> (w601:T15)
            n232 = for {
              shift-right: [w621] -> w599
              shift-left: w602 -> [w625]
              tunnel: w601 -> [w623] mode=indexing
              n233 = Unbundle By Name(w623) -> ("UDP ref"=w622:refnum<k16>)
              n234 = UDP Close(connection ID=w622, 8:w625) -> (error out=w624:errorcluster)  [unwired: 1 out]
              n235 = call <vilib>:"Clear Errors.vi"("error in (no error)"=w624) -> ("error out"=w621:errorcluster)  [unwired: 5 in, 1 out]
            }
            n236 = call "Main - Manual Control Deamon Ref (FGV).vi"("Action"=FGV_States."Read", "error in"=w599) -> ("error out"=w598:errorcluster, "Ref out"=w597:refnum<vi>[])  [unwired: 7 in, 1 out]
            n237 = call "General - Exit eFGV.vi"("eFGV States"=eFGV_States."Write", "error in (no error)"=w598, "Exit In"=TRUE) -> ("error out"=w611:errorcluster)  [unwired: 6 in, 2 out]
            n238 = call "Runtest - Deamon Ref (FGV).vi"("Action"=FGV_States."Read", "error in"=w611) -> ("error out"=w614:errorcluster, "Ref out"=w596:refnum<vi>[])  [unwired: 7 in, 1 out]
            n239 = Build Array (concatenate)(w613, w597, w596) -> (w612:refnum<vi>[])
            n240 = for {
              tunnel: w612 -> [w631] mode=indexing
              shift-right: [w632] -> w605
              shift-left: w614 -> [w634]
              n241 = invoke class="VI" method="Abort VI"(reference=w631, error in=w634) -> (error out=w633:errorcluster)  [unwired: 1 in, 2 out]
              n242 = call <vilib>:"Clear Errors.vi"("error in (no error)"=w633) -> ("error out"=w632:errorcluster)  [unwired: 5 in, 1 out]
            }
            n243 = control-ref of="This VI"() -> (w610:refnum<vi>)
            n244 = invoke class="VI" method="FP.Close"(reference=w610, error in=w605) -> (reference out=w607:refnum<vi>, error out=w609:errorcluster)  [unwired: 1 in, 1 out]
            n245 = call <vilib>:"Unset Busy.vi"("error in (no error)"=w609, "VI reference (current VI)"=w607) -> ("error out"=w608:errorcluster)  [unwired: 9 in]
          }
        }
      }
      frame Error {
        n246 = call <vilib>:"Clear Errors.vi"("error in (no error)"=w640) -> ("error out"=w637:errorcluster)  [unwired: 5 in, 1 out]
        n247 = Wait (ms)(milliseconds to wait=u32 100) -> ()  [unwired: 1 out]
      }
    }
  }
  n248 = case shown="No Error" w8 {
    frame No Error {
      w651 = string[] [] ("SN")
      n249 = global write "Global - Done.vi" "Done"(bool[] [FALSE, FALSE, FALSE, FALSE, FALSE, FALSE, FALSE, FALSE, FALSE, FALSE, FALSE, FALSE, FALSE, FALSE, FALSE, FALSE] ("Done")) -> ()
      n250 = global write "Global - Channel.vi" "Data"(T18 [{"Channels"={"Ch1"=0.0, "Ch2"=0.0, "Ch3"=0.0, "Ch4"=0.0, "Ch5"=0.0, "Ch6"=0.0, "Ch7"=0.0, "Ch8"=0.0, "Ch9"=0.0, "Ch10"=0.0, "Ch11"=0.0, "Ch12"=0.0, "Ch13"=0.0, "Ch14"=0.0, "Ch15"=0.0, "Ch16"=0.0}, "Event"=0, "Status"=0}, {"Channels"={"Ch1"=0.0, "Ch2"=0.0, "Ch3"=0.0, "Ch4"=0.0, "Ch5"=0.0, "Ch6"=0.0, "Ch7"=0.0, "Ch8"=0.0, "Ch9"=0.0, "Ch10"=0.0, "Ch11"=0.0, "Ch12"=0.0, "Ch13"=0.0, "Ch14"=0.0, "Ch15"=0.0, "Ch16"=0.0}, "Event"=0, "Status"=0}, {"Channels"={"Ch1"=0.0, "Ch2"=0.0, "Ch3"=0.0, "Ch4"=0.0, "Ch5"=0.0, "Ch6"=0.0, "Ch7"=0.0, "Ch8"=0.0, "Ch9"=0.0, "Ch10"=0.0, "Ch11"=0.0, "Ch12"=0.0, "Ch13"=0.0, "Ch14"=0.0, "Ch15"=0.0, "Ch16"=0.0}, "Event"=0, "Status"=0}, {"Channels"={"Ch1"=0.0, "Ch2"=0.0, "Ch3"=0.0, "Ch4"=0.0, "Ch5"=0.0, "Ch6"=0.0, "Ch7"=0.0, "Ch8"=0.0, "Ch9"=0.0, "Ch10"=0.0, "Ch11"=0.0, "Ch12"=0.0, "Ch13"=0.0, "Ch14"=0.0, "Ch15"=0.0, "Ch16"=0.0}, "Event"=0, "Status"=0}, {"Channels"={"Ch1"=0.0, "Ch2"=0.0, "Ch3"=0.0, "Ch4"=0.0, "Ch5"=0.0, "Ch6"=0.0, "Ch7"=0.0, "Ch8"=0.0, "Ch9"=0.0, "Ch10"=0.0, "Ch11"=0.0, "Ch12"=0.0, "Ch13"=0.0, "Ch14"=0.0, "Ch15"=0.0, "Ch16"=0.0}, "Event"=0, "Status"=0}, {"Channels"={"Ch1"=0.0, "Ch2"=0.0, "Ch3"=0.0, "Ch4"=0.0, "Ch5"=0.0, "Ch6"=0.0, "Ch7"=0.0, "Ch8"=0.0, "Ch9"=0.0, "Ch10"=0.0, "Ch11"=0.0, "Ch12"=0.0, "Ch13"=0.0, "Ch14"=0.0, "Ch15"=0.0, "Ch16"=0.0}, "Event"=0, "Status"=0}, {"Channels"={"Ch1"=0.0, "Ch2"=0.0, "Ch3"=0.0, "Ch4"=0.0, "Ch5"=0.0, "Ch6"=0.0, "Ch7"=0.0, "Ch8"=0.0, "Ch9"=0.0, "Ch10"=0.0, "Ch11"=0.0, "Ch12"=0.0, "Ch13"=0.0, "Ch14"=0.0, "Ch15"=0.0, "Ch16"=0.0}, "Event"=0, "Status"=0}, {"Channels"={"Ch1"=0.0, "Ch2"=0.0, "Ch3"=0.0, "Ch4"=0.0, "Ch5"=0.0, "Ch6"=0.0, "Ch7"=0.0, "Ch8"=0.0, "Ch9"=0.0, "Ch10"=0.0, "Ch11"=0.0, "Ch12"=0.0, "Ch13"=0.0, "Ch14"=0.0, "Ch15"=0.0, "Ch16"=0.0}, "Event"=0, "Status"=0}, {"Channels"={"Ch1"=0.0, "Ch2"=0.0, "Ch3"=0.0, "Ch4"=0.0, "Ch5"=0.0, "Ch6"=0.0, "Ch7"=0.0, "Ch8"=0.0, "Ch9"=0.0, "Ch10"=0.0, "Ch11"=0.0, "Ch12"=0.0, "Ch13"=0.0, "Ch14"=0.0, "Ch15"=0.0, "Ch16"=0.0}, "Event"=0, "Status"=0}, {"Channels"={"Ch1"=0.0, "Ch2"=0.0, "Ch3"=0.0, "Ch4"=0.0, "Ch5"=0.0, "Ch6"=0.0, "Ch7"=0.0, "Ch8"=0.0, "Ch9"=0.0, "Ch10"=0.0, "Ch11"=0.0, "Ch12"=0.0, "Ch13"=0.0, "Ch14"=0.0, "Ch15"=0.0, "Ch16"=0.0}, "Event"=0, "Status"=0}, {"Channels"={"Ch1"=0.0, "Ch2"=0.0, "Ch3"=0.0, "Ch4"=0.0, "Ch5"=0.0, "Ch6"=0.0, "Ch7"=0.0, "Ch8"=0.0, "Ch9"=0.0, "Ch10"=0.0, "Ch11"=0.0, "Ch12"=0.0, "Ch13"=0.0, "Ch14"=0.0, "Ch15"=0.0, "Ch16"=0.0}, "Event"=0, "Status"=0}, {"Channels"={"Ch1"=0.0, "Ch2"=0.0, "Ch3"=0.0, "Ch4"=0.0, "Ch5"=0.0, "Ch6"=0.0, "Ch7"=0.0, "Ch8"=0.0, "Ch9"=0.0, "Ch10"=0.0, "Ch11"=0.0, "Ch12"=0.0, "Ch13"=0.0, "Ch14"=0.0, "Ch15"=0.0, "Ch16"=0.0}, "Event"=0, "Status"=0}, {"Channels"={"Ch1"=0.0, "Ch2"=0.0, "Ch3"=0.0, "Ch4"=0.0, "Ch5"=0.0, "Ch6"=0.0, "Ch7"=0.0, "Ch8"=0.0, "Ch9"=0.0, "Ch10"=0.0, "Ch11"=0.0, "Ch12"=0.0, "Ch13"=0.0, "Ch14"=0.0, "Ch15"=0.0, "Ch16"=0.0}, "Event"=0, "Status"=0}, {"Channels"={"Ch1"=0.0, "Ch2"=0.0, "Ch3"=0.0, "Ch4"=0.0, "Ch5"=0.0, "Ch6"=0.0, "Ch7"=0.0, "Ch8"=0.0, "Ch9"=0.0, "Ch10"=0.0, "Ch11"=0.0, "Ch12"=0.0, "Ch13"=0.0, "Ch14"=0.0, "Ch15"=0.0, "Ch16"=0.0}, "Event"=0, "Status"=0}, {"Channels"={"Ch1"=0.0, "Ch2"=0.0, "Ch3"=0.0, "Ch4"=0.0, "Ch5"=0.0, "Ch6"=0.0, "Ch7"=0.0, "Ch8"=0.0, "Ch9"=0.0, "Ch10"=0.0, "Ch11"=0.0, "Ch12"=0.0, "Ch13"=0.0, "Ch14"=0.0, "Ch15"=0.0, "Ch16"=0.0}, "Event"=0, "Status"=0}, {"Channels"={"Ch1"=0.0, "Ch2"=0.0, "Ch3"=0.0, "Ch4"=0.0, "Ch5"=0.0, "Ch6"=0.0, "Ch7"=0.0, "Ch8"=0.0, "Ch9"=0.0, "Ch10"=0.0, "Ch11"=0.0, "Ch12"=0.0, "Ch13"=0.0, "Ch14"=0.0, "Ch15"=0.0, "Ch16"=0.0}, "Event"=0, "Status"=0}] ("Data")) -> ()
      n251 = global write "Global - Data UDP.vi" "Channels"(T19 {"Ch1"=0.0, "Ch2"=0.0, "Ch3"=0.0, "Ch4"=0.0, "Ch5"=0.0, "Ch6"=0.0, "Ch7"=0.0, "Ch8"=0.0, "Ch9"=0.0, "Ch10"=0.0, "Ch11"=0.0, "Ch12"=0.0, "Ch13"=0.0, "Ch14"=0.0, "Ch15"=0.0, "Ch16"=0.0} ("Channels")) -> ()
      n252 = global write "Global - PID.vi" "PID"(T22 [{"SP"=0.0, "PV"=0.0, "kP"=0.0, "kI"=0.0, "kD"=0.0, "FF"=0.0, "Err Band"=0.0, "Max"=0, "Min"=0, "Ts"=0, "Out"=0, "Mode"=0}, {"SP"=0.0, "PV"=0.0, "kP"=0.0, "kI"=0.0, "kD"=0.0, "FF"=0.0, "Err Band"=0.0, "Max"=0, "Min"=0, "Ts"=0, "Out"=0, "Mode"=0}, {"SP"=0.0, "PV"=0.0, "kP"=0.0, "kI"=0.0, "kD"=0.0, "FF"=0.0, "Err Band"=0.0, "Max"=0, "Min"=0, "Ts"=0, "Out"=0, "Mode"=0}, {"SP"=0.0, "PV"=0.0, "kP"=0.0, "kI"=0.0, "kD"=0.0, "FF"=0.0, "Err Band"=0.0, "Max"=0, "Min"=0, "Ts"=0, "Out"=0, "Mode"=0}, {"SP"=0.0, "PV"=0.0, "kP"=0.0, "kI"=0.0, "kD"=0.0, "FF"=0.0, "Err Band"=0.0, "Max"=0, "Min"=0, "Ts"=0, "Out"=0, "Mode"=0}, {"SP"=0.0, "PV"=0.0, "kP"=0.0, "kI"=0.0, "kD"=0.0, "FF"=0.0, "Err Band"=0.0, "Max"=0, "Min"=0, "Ts"=0, "Out"=0, "Mode"=0}, {"SP"=0.0, "PV"=0.0, "kP"=0.0, "kI"=0.0, "kD"=0.0, "FF"=0.0, "Err Band"=0.0, "Max"=0, "Min"=0, "Ts"=0, "Out"=0, "Mode"=0}, {"SP"=0.0, "PV"=0.0, "kP"=0.0, "kI"=0.0, "kD"=0.0, "FF"=0.0, "Err Band"=0.0, "Max"=0, "Min"=0, "Ts"=0, "Out"=0, "Mode"=0}, {"SP"=0.0, "PV"=0.0, "kP"=0.0, "kI"=0.0, "kD"=0.0, "FF"=0.0, "Err Band"=0.0, "Max"=0, "Min"=0, "Ts"=0, "Out"=0, "Mode"=0}, {"SP"=0.0, "PV"=0.0, "kP"=0.0, "kI"=0.0, "kD"=0.0, "FF"=0.0, "Err Band"=0.0, "Max"=0, "Min"=0, "Ts"=0, "Out"=0, "Mode"=0}, {"SP"=0.0, "PV"=0.0, "kP"=0.0, "kI"=0.0, "kD"=0.0, "FF"=0.0, "Err Band"=0.0, "Max"=0, "Min"=0, "Ts"=0, "Out"=0, "Mode"=0}, {"SP"=0.0, "PV"=0.0, "kP"=0.0, "kI"=0.0, "kD"=0.0, "FF"=0.0, "Err Band"=0.0, "Max"=0, "Min"=0, "Ts"=0, "Out"=0, "Mode"=0}, {"SP"=0.0, "PV"=0.0, "kP"=0.0, "kI"=0.0, "kD"=0.0, "FF"=0.0, "Err Band"=0.0, "Max"=0, "Min"=0, "Ts"=0, "Out"=0, "Mode"=0}, {"SP"=0.0, "PV"=0.0, "kP"=0.0, "kI"=0.0, "kD"=0.0, "FF"=0.0, "Err Band"=0.0, "Max"=0, "Min"=0, "Ts"=0, "Out"=0, "Mode"=0}, {"SP"=0.0, "PV"=0.0, "kP"=0.0, "kI"=0.0, "kD"=0.0, "FF"=0.0, "Err Band"=0.0, "Max"=0, "Min"=0, "Ts"=0, "Out"=0, "Mode"=0}, {"SP"=0.0, "PV"=0.0, "kP"=0.0, "kI"=0.0, "kD"=0.0, "FF"=0.0, "Err Band"=0.0, "Max"=0, "Min"=0, "Ts"=0, "Out"=0, "Mode"=0}] ("PID")) -> ()
      n253 = global write "Global - Device.vi" "Device"(w651) -> ()
      n254 = global write "Global - Handle.vi" "Handle"(T15 [] ("Handle")) -> ()
      n255 = global write "Global - Test.vi" "Test"(T20 [{"Target Load"=0.0, "Target Disp"=0.0, "Rate"=0.0, "Speed"=0.0}, {"Target Load"=0.0, "Target Disp"=0.0, "Rate"=0.0, "Speed"=0.0}, {"Target Load"=0.0, "Target Disp"=0.0, "Rate"=0.0, "Speed"=0.0}, {"Target Load"=0.0, "Target Disp"=0.0, "Rate"=0.0, "Speed"=0.0}, {"Target Load"=0.0, "Target Disp"=0.0, "Rate"=0.0, "Speed"=0.0}, {"Target Load"=0.0, "Target Disp"=0.0, "Rate"=0.0, "Speed"=0.0}, {"Target Load"=0.0, "Target Disp"=0.0, "Rate"=0.0, "Speed"=0.0}, {"Target Load"=0.0, "Target Disp"=0.0, "Rate"=0.0, "Speed"=0.0}, {"Target Load"=0.0, "Target Disp"=0.0, "Rate"=0.0, "Speed"=0.0}, {"Target Load"=0.0, "Target Disp"=0.0, "Rate"=0.0, "Speed"=0.0}, {"Target Load"=0.0, "Target Disp"=0.0, "Rate"=0.0, "Speed"=0.0}, {"Target Load"=0.0, "Target Disp"=0.0, "Rate"=0.0, "Speed"=0.0}, {"Target Load"=0.0, "Target Disp"=0.0, "Rate"=0.0, "Speed"=0.0}, {"Target Load"=0.0, "Target Disp"=0.0, "Rate"=0.0, "Speed"=0.0}, {"Target Load"=0.0, "Target Disp"=0.0, "Rate"=0.0, "Speed"=0.0}, {"Target Load"=0.0, "Target Disp"=0.0, "Rate"=0.0, "Speed"=0.0}] ("Test")) -> ()
      n256 = global write "Global - System.vi" "System"(T21 [{"Out Type"=0, "Inverse"=0, "Monitor"=0, "Reserve"=0, "ACC Time"=0, "Pulse Rev"=0, "Stroke"=0, "Auto Off"=0, "Gear Ratio"=0.0, "Pitch"=0.0, "Max Speed"=0, "Jog Speed"=0, "Disp Coff"=0.0, "Max Load"=0}, {"Out Type"=0, "Inverse"=0, "Monitor"=0, "Reserve"=0, "ACC Time"=0, "Pulse Rev"=0, "Stroke"=0, "Auto Off"=0, "Gear Ratio"=0.0, "Pitch"=0.0, "Max Speed"=0, "Jog Speed"=0, "Disp Coff"=0.0, "Max Load"=0}, {"Out Type"=0, "Inverse"=0, "Monitor"=0, "Reserve"=0, "ACC Time"=0, "Pulse Rev"=0, "Stroke"=0, "Auto Off"=0, "Gear Ratio"=0.0, "Pitch"=0.0, "Max Speed"=0, "Jog Speed"=0, "Disp Coff"=0.0, "Max Load"=0}, {"Out Type"=0, "Inverse"=0, "Monitor"=0, "Reserve"=0, "ACC Time"=0, "Pulse Rev"=0, "Stroke"=0, "Auto Off"=0, "Gear Ratio"=0.0, "Pitch"=0.0, "Max Speed"=0, "Jog Speed"=0, "Disp Coff"=0.0, "Max Load"=0}, {"Out Type"=0, "Inverse"=0, "Monitor"=0, "Reserve"=0, "ACC Time"=0, "Pulse Rev"=0, "Stroke"=0, "Auto Off"=0, "Gear Ratio"=0.0, "Pitch"=0.0, "Max Speed"=0, "Jog Speed"=0, "Disp Coff"=0.0, "Max Load"=0}, {"Out Type"=0, "Inverse"=0, "Monitor"=0, "Reserve"=0, "ACC Time"=0, "Pulse Rev"=0, "Stroke"=0, "Auto Off"=0, "Gear Ratio"=0.0, "Pitch"=0.0, "Max Speed"=0, "Jog Speed"=0, "Disp Coff"=0.0, "Max Load"=0}, {"Out Type"=0, "Inverse"=0, "Monitor"=0, "Reserve"=0, "ACC Time"=0, "Pulse Rev"=0, "Stroke"=0, "Auto Off"=0, "Gear Ratio"=0.0, "Pitch"=0.0, "Max Speed"=0, "Jog Speed"=0, "Disp Coff"=0.0, "Max Load"=0}, {"Out Type"=0, "Inverse"=0, "Monitor"=0, "Reserve"=0, "ACC Time"=0, "Pulse Rev"=0, "Stroke"=0, "Auto Off"=0, "Gear Ratio"=0.0, "Pitch"=0.0, "Max Speed"=0, "Jog Speed"=0, "Disp Coff"=0.0, "Max Load"=0}, {"Out Type"=0, "Inverse"=0, "Monitor"=0, "Reserve"=0, "ACC Time"=0, "Pulse Rev"=0, "Stroke"=0, "Auto Off"=0, "Gear Ratio"=0.0, "Pitch"=0.0, "Max Speed"=0, "Jog Speed"=0, "Disp Coff"=0.0, "Max Load"=0}, {"Out Type"=0, "Inverse"=0, "Monitor"=0, "Reserve"=0, "ACC Time"=0, "Pulse Rev"=0, "Stroke"=0, "Auto Off"=0, "Gear Ratio"=0.0, "Pitch"=0.0, "Max Speed"=0, "Jog Speed"=0, "Disp Coff"=0.0, "Max Load"=0}, {"Out Type"=0, "Inverse"=0, "Monitor"=0, "Reserve"=0, "ACC Time"=0, "Pulse Rev"=0, "Stroke"=0, "Auto Off"=0, "Gear Ratio"=0.0, "Pitch"=0.0, "Max Speed"=0, "Jog Speed"=0, "Disp Coff"=0.0, "Max Load"=0}, {"Out Type"=0, "Inverse"=0, "Monitor"=0, "Reserve"=0, "ACC Time"=0, "Pulse Rev"=0, "Stroke"=0, "Auto Off"=0, "Gear Ratio"=0.0, "Pitch"=0.0, "Max Speed"=0, "Jog Speed"=0, "Disp Coff"=0.0, "Max Load"=0}, {"Out Type"=0, "Inverse"=0, "Monitor"=0, "Reserve"=0, "ACC Time"=0, "Pulse Rev"=0, "Stroke"=0, "Auto Off"=0, "Gear Ratio"=0.0, "Pitch"=0.0, "Max Speed"=0, "Jog Speed"=0, "Disp Coff"=0.0, "Max Load"=0}, {"Out Type"=0, "Inverse"=0, "Monitor"=0, "Reserve"=0, "ACC Time"=0, "Pulse Rev"=0, "Stroke"=0, "Auto Off"=0, "Gear Ratio"=0.0, "Pitch"=0.0, "Max Speed"=0, "Jog Speed"=0, "Disp Coff"=0.0, "Max Load"=0}, {"Out Type"=0, "Inverse"=0, "Monitor"=0, "Reserve"=0, "ACC Time"=0, "Pulse Rev"=0, "Stroke"=0, "Auto Off"=0, "Gear Ratio"=0.0, "Pitch"=0.0, "Max Speed"=0, "Jog Speed"=0, "Disp Coff"=0.0, "Max Load"=0}, {"Out Type"=0, "Inverse"=0, "Monitor"=0, "Reserve"=0, "ACC Time"=0, "Pulse Rev"=0, "Stroke"=0, "Auto Off"=0, "Gear Ratio"=0.0, "Pitch"=0.0, "Max Speed"=0, "Jog Speed"=0, "Disp Coff"=0.0, "Max Load"=0}] ("System")) -> ()
      n257 = global write "Global - IP Address.vi" "IP"(w651) -> ()
      n258 = global write "Global - Unit.vi" "Unit"(T24 [{"Name"=[], "Unit"=[], "Decimal Point"=[], "Ch Log"=[], "H Alarm"=[], "L Alarm"=[], "H Limit"=[], "L Limit"=[], "Filter"=[], "Gain"=[], "Calib Type"=[]}, {"Name"=[], "Unit"=[], "Decimal Point"=[], "Ch Log"=[], "H Alarm"=[], "L Alarm"=[], "H Limit"=[], "L Limit"=[], "Filter"=[], "Gain"=[], "Calib Type"=[]}, {"Name"=[], "Unit"=[], "Decimal Point"=[], "Ch Log"=[], "H Alarm"=[], "L Alarm"=[], "H Limit"=[], "L Limit"=[], "Filter"=[], "Gain"=[], "Calib Type"=[]}, {"Name"=[], "Unit"=[], "Decimal Point"=[], "Ch Log"=[], "H Alarm"=[], "L Alarm"=[], "H Limit"=[], "L Limit"=[], "Filter"=[], "Gain"=[], "Calib Type"=[]}, {"Name"=[], "Unit"=[], "Decimal Point"=[], "Ch Log"=[], "H Alarm"=[], "L Alarm"=[], "H Limit"=[], "L Limit"=[], "Filter"=[], "Gain"=[], "Calib Type"=[]}, {"Name"=[], "Unit"=[], "Decimal Point"=[], "Ch Log"=[], "H Alarm"=[], "L Alarm"=[], "H Limit"=[], "L Limit"=[], "Filter"=[], "Gain"=[], "Calib Type"=[]}, {"Name"=[], "Unit"=[], "Decimal Point"=[], "Ch Log"=[], "H Alarm"=[], "L Alarm"=[], "H Limit"=[], "L Limit"=[], "Filter"=[], "Gain"=[], "Calib Type"=[]}, {"Name"=[], "Unit"=[], "Decimal Point"=[], "Ch Log"=[], "H Alarm"=[], "L Alarm"=[], "H Limit"=[], "L Limit"=[], "Filter"=[], "Gain"=[], "Calib Type"=[]}, {"Name"=[], "Unit"=[], "Decimal Point"=[], "Ch Log"=[], "H Alarm"=[], "L Alarm"=[], "H Limit"=[], "L Limit"=[], "Filter"=[], "Gain"=[], "Calib Type"=[]}, {"Name"=[], "Unit"=[], "Decimal Point"=[], "Ch Log"=[], "H Alarm"=[], "L Alarm"=[], "H Limit"=[], "L Limit"=[], "Filter"=[], "Gain"=[], "Calib Type"=[]}, {"Name"=[], "Unit"=[], "Decimal Point"=[], "Ch Log"=[], "H Alarm"=[], "L Alarm"=[], "H Limit"=[], "L Limit"=[], "Filter"=[], "Gain"=[], "Calib Type"=[]}, {"Name"=[], "Unit"=[], "Decimal Point"=[], "Ch Log"=[], "H Alarm"=[], "L Alarm"=[], "H Limit"=[], "L Limit"=[], "Filter"=[], "Gain"=[], "Calib Type"=[]}, {"Name"=[], "Unit"=[], "Decimal Point"=[], "Ch Log"=[], "H Alarm"=[], "L Alarm"=[], "H Limit"=[], "L Limit"=[], "Filter"=[], "Gain"=[], "Calib Type"=[]}, {"Name"=[], "Unit"=[], "Decimal Point"=[], "Ch Log"=[], "H Alarm"=[], "L Alarm"=[], "H Limit"=[], "L Limit"=[], "Filter"=[], "Gain"=[], "Calib Type"=[]}, {"Name"=[], "Unit"=[], "Decimal Point"=[], "Ch Log"=[], "H Alarm"=[], "L Alarm"=[], "H Limit"=[], "L Limit"=[], "Filter"=[], "Gain"=[], "Calib Type"=[]}, {"Name"=[], "Unit"=[], "Decimal Point"=[], "Ch Log"=[], "H Alarm"=[], "L Alarm"=[], "H Limit"=[], "L Limit"=[], "Filter"=[], "Gain"=[], "Calib Type"=[]}] ("Unit")) -> ()
      n259 = global write "Global - ADC.vi" "ADC"(T23 [{"Active Ch"=[], "Filter Type"=0, "Post Filter"=[], "Gain"=[], "FS"=0, "IntOC"=0, "IntFC"=0, "SysOC"=0, "Cofficient"=[], "K"=[], "Max"=0}, {"Active Ch"=[], "Filter Type"=0, "Post Filter"=[], "Gain"=[], "FS"=0, "IntOC"=0, "IntFC"=0, "SysOC"=0, "Cofficient"=[], "K"=[], "Max"=0}, {"Active Ch"=[], "Filter Type"=0, "Post Filter"=[], "Gain"=[], "FS"=0, "IntOC"=0, "IntFC"=0, "SysOC"=0, "Cofficient"=[], "K"=[], "Max"=0}, {"Active Ch"=[], "Filter Type"=0, "Post Filter"=[], "Gain"=[], "FS"=0, "IntOC"=0, "IntFC"=0, "SysOC"=0, "Cofficient"=[], "K"=[], "Max"=0}, {"Active Ch"=[], "Filter Type"=0, "Post Filter"=[], "Gain"=[], "FS"=0, "IntOC"=0, "IntFC"=0, "SysOC"=0, "Cofficient"=[], "K"=[], "Max"=0}, {"Active Ch"=[], "Filter Type"=0, "Post Filter"=[], "Gain"=[], "FS"=0, "IntOC"=0, "IntFC"=0, "SysOC"=0, "Cofficient"=[], "K"=[], "Max"=0}, {"Active Ch"=[], "Filter Type"=0, "Post Filter"=[], "Gain"=[], "FS"=0, "IntOC"=0, "IntFC"=0, "SysOC"=0, "Cofficient"=[], "K"=[], "Max"=0}, {"Active Ch"=[], "Filter Type"=0, "Post Filter"=[], "Gain"=[], "FS"=0, "IntOC"=0, "IntFC"=0, "SysOC"=0, "Cofficient"=[], "K"=[], "Max"=0}, {"Active Ch"=[], "Filter Type"=0, "Post Filter"=[], "Gain"=[], "FS"=0, "IntOC"=0, "IntFC"=0, "SysOC"=0, "Cofficient"=[], "K"=[], "Max"=0}, {"Active Ch"=[], "Filter Type"=0, "Post Filter"=[], "Gain"=[], "FS"=0, "IntOC"=0, "IntFC"=0, "SysOC"=0, "Cofficient"=[], "K"=[], "Max"=0}, {"Active Ch"=[], "Filter Type"=0, "Post Filter"=[], "Gain"=[], "FS"=0, "IntOC"=0, "IntFC"=0, "SysOC"=0, "Cofficient"=[], "K"=[], "Max"=0}, {"Active Ch"=[], "Filter Type"=0, "Post Filter"=[], "Gain"=[], "FS"=0, "IntOC"=0, "IntFC"=0, "SysOC"=0, "Cofficient"=[], "K"=[], "Max"=0}, {"Active Ch"=[], "Filter Type"=0, "Post Filter"=[], "Gain"=[], "FS"=0, "IntOC"=0, "IntFC"=0, "SysOC"=0, "Cofficient"=[], "K"=[], "Max"=0}, {"Active Ch"=[], "Filter Type"=0, "Post Filter"=[], "Gain"=[], "FS"=0, "IntOC"=0, "IntFC"=0, "SysOC"=0, "Cofficient"=[], "K"=[], "Max"=0}, {"Active Ch"=[], "Filter Type"=0, "Post Filter"=[], "Gain"=[], "FS"=0, "IntOC"=0, "IntFC"=0, "SysOC"=0, "Cofficient"=[], "K"=[], "Max"=0}, {"Active Ch"=[], "Filter Type"=0, "Post Filter"=[], "Gain"=[], "FS"=0, "IntOC"=0, "IntFC"=0, "SysOC"=0, "Cofficient"=[], "K"=[], "Max"=0}] ("ADC")) -> ()
      n260 = global write "Global - Comport.vi" "Port"(string[] [] ("Comport")) -> ()
    }
    frame Error {
    }
  }
